vi "Session handler.vi"(0 "Loop data":T14={"Persistent"={"Last file"=path "", "Last user"="", "Users"=[]}, "Temp handle"={"Connected"=FALSE, "Temp ctrl"={"Gain (P)"=0.0, "Reset (I)"=0.0, "Rate (D)"=0.0, "Stabilization rate"=0.0, "Stabilization delta"=0.0, "Type"=enum."Lake Shore 325", "Custom temp ctrl"={"VISA resource name"=""}, "Lakeshore 325"={"VISA name"="", "Loop"=0, "Heater Range"=1, "Heater Resistance"=0, "Sample sensor"=0, "Fast sensor"=0, "Slow sensor"=0}, "Lakeshore 331"={"VISA name"="", "Loop"=1, "Heater Range"=0, "Sample sensor"=0, "Fast sensor"=0, "Slow sensor"=0}, "Lakeshore 332"={"VISA name"="", "Loop"=1, "Heater Range"=0, "Sample sensor"=0, "Fast sensor"=0, "Slow sensor"=0}, "Lakeshore 335"={"VISA name"="", "Loop"=1, "Sample sensor"=0, "Fast sensor"=0, "Slow sensor"=0, "Heater Range"=0, "Output mode"=enum."Off"}, "Lakeshore 336"={"VISA name"="", "Loop"=1, "Output mode"=enum."Off", "Max current"=1.0, "Heater resistance"=1, "Sample sensor"=1, "Slow sensor"=1, "Fast sensor"=1}}}, "Paths"={"Manual"=path "", "Settings"=path "", "Persistent"=path "", "Work dir."=path ""}, "Settings"={"MFIA"={"Address"="", "Use compensation"=TRUE, "Shut down gracefully"=FALSE}, "Temp ctrl"={"Gain (P)"=0.0, "Reset (I)"=0.0, "Rate (D)"=0.0, "Stabilization rate"=0.0, "Stabilization delta"=0.0, "Type"=enum."Lake Shore 325", "Custom temp ctrl"={"VISA resource name"=""}, "Lakeshore 325"={"VISA name"="", "Loop"=0, "Heater Range"=1, "Heater Resistance"=0, "Sample sensor"=0, "Fast sensor"=0, "Slow sensor"=0}, "Lakeshore 331"={"VISA name"="", "Loop"=1, "Heater Range"=0, "Sample sensor"=0, "Fast sensor"=0, "Slow sensor"=0}, "Lakeshore 332"={"VISA name"="", "Loop"=1, "Heater Range"=0, "Sample sensor"=0, "Fast sensor"=0, "Slow sensor"=0}, "Lakeshore 335"={"VISA name"="", "Loop"=1, "Sample sensor"=0, "Fast sensor"=0, "Slow sensor"=0, "Heater Range"=0, "Output mode"=enum."Off"}, "Lakeshore 336"={"VISA name"="", "Loop"=1, "Output mode"=enum."Off", "Max current"=1.0, "Heater resistance"=1, "Sample sensor"=1, "Slow sensor"=1, "Fast sensor"=1}}, "Source-meter"={"Type"=enum."Custom", "Custom source-meter"={"VISA resource name"=""}, "Keithley 2600"={"VISA name"="", "Ignore ID Query"=FALSE, "SMU"=enum."Channel A"}, "Keithley 2400 Series"={"VISA name"="", "Ignore ID Query"=FALSE}}, "Other"={"Enable OriginLab"=FALSE, "Reader mode"=FALSE, "Auto-save"=FALSE}, "Defaults"={"IV properties"={"T"=0.0, "Vstart"=-0.5, "Vstop"=0.5, "Vpoints"=10.0, "Settling"=0.01, "I limit"=0.1, "Log mapping"=FALSE, "Averaging"=0.0}, "CV properties"={"T"=0.0, "Vstart"=-0.5, "Vstop"=0.5, "Vpoints"=10.0, "Precision"=enum."Normal", "Test signal"=0.01, "Auto I range"=FALSE, "Test frequency"=100000.0, "I range"=-2.0, "V range"=10.0, "Log mapping"=FALSE, "Rel perm"=0.0, "Area"=0.0, "Equivalent circuit model"=0}, "DLTS properties"={"Tstart"=0.0, "Instant start"=FALSE, "Tstop"=0.0, "T rate"=0.0, "Test signal"=0.0, "Test frequency"=0.0, "Bandwidth"=0.0, "Averaging"=0.0, "Vbias"=0.0, "Vpulse"=0.0, "pulse length"=0.0, "Pulse 2"=FALSE, "Vpulse 2"=0.0, "pulse length 2"=0.0, "I range"=-2.0, "V range"=10.0, "Emission rate"=[], "Sampling rate"=0.0, "Acq. delay"=0.0, "Filter order"=0, "Equivalent circuit model"=0}, "LDLTS properties"={"T"=0.0, "Test signal"=0.0, "Test frequency"=0.0, "Bandwidth"=0.0, "Averaging"=0.0, "Vbias"=0.0, "Vpulse"=0.0, "pulse length"=0.0, "Pulse 2"=FALSE, "Vpulse 2"=0.0, "pulse length 2"=0.0, "I range"=-2.0, "V range"=10.0, "Sampling rate"=0.0, "Acq. delay"=0.0, "Sampling time"=0.0, "Filter order"=0, "Equivalent circuit model"=0}}}, "Software version"=0.0, "MFIA handle"={"ziHandle"={"handleValid"=FALSE, "Conn"=0, "Path Prefix"="", "Handle"=0, "Connected"=FALSE, "Clockbase(s)"=0.0}, "Selected device"="", "ziModHandle"={"handleValid"=FALSE, "Conn"=0, "ModHandle"=0, "moduleID"="", "Path Prefix"=""}}, "Source-meter handle"={"Connected"=FALSE, "Source-meter"={"Type"=enum."Custom", "Custom source-meter"={"VISA resource name"=""}, "Keithley 2600"={"VISA name"="", "Ignore ID Query"=FALSE, "SMU"=enum."Channel A"}, "Keithley 2400 Series"={"VISA name"="", "Ignore ID Query"=FALSE}}}} {"MFIA handle"."ziModHandle"."ModHandle" format="0x%08x"; "MFIA handle"."ziModHandle"."Conn" format="0x%08x"; "MFIA handle"."ziHandle"."Handle" format="0x%08x"; "MFIA handle"."ziHandle"."Conn" format="0x%08x"; "Settings"."Defaults"."LDLTS properties"."Equivalent circuit model" items=["Rp || Cp", "Rs + Cs", "Rs + Ls", "G B", "D Cs", "Q Cs", "D Ls", "Q Ls", "Rp || Lp", "D Cp"]; "Settings"."Defaults"."LDLTS properties"."Filter order" min=0 max=8 step=1; "Settings"."Defaults"."LDLTS properties"."Sampling rate" items=["13k"=13392.857422, "27k"=26785.714844, "54k"=53571.429687, "107k"=107142.859375]; "Settings"."Defaults"."LDLTS properties"."V range" items=["10mV"=0.01, "100mV"=0.1, "1V"=1.0, "10V"=10.0]; "Settings"."Defaults"."LDLTS properties"."I range" items=["100nA"=-7.0, "1µA"=-6.0, "10µA"=-5.0, "100µA"=-4.0, "1mA"=-3.0, "10mA"=-2.0]; "Settings"."Defaults"."DLTS properties"."Equivalent circuit model" items=["Rp || Cp", "Rs + Cs", "Rs + Ls", "G B", "D Cs", "Q Cs", "D Ls", "Q Ls", "Rp || Lp", "D Cp"]; "Settings"."Defaults"."DLTS properties"."Filter order" min=0 max=8 step=1; "Settings"."Defaults"."DLTS properties"."Sampling rate" items=["13k"=13392.857422, "27k"=26785.714844, "54k"=53571.429687, "107k"=107142.859375]; "Settings"."Defaults"."DLTS properties"."V range" items=["10mV"=0.01, "100mV"=0.1, "1V"=1.0, "10V"=10.0]; "Settings"."Defaults"."DLTS properties"."I range" items=["10mV"=0.01, "100mV"=0.1, "1V"=1.0, "10V"=10.0]; "Settings"."Defaults"."CV properties"."Equivalent circuit model" items=["Rp || Cp", "Rs + Cs", "Rs + Ls", "G B", "D Cs", "Q Cs", "D Ls", "Q Ls", "Rp || Lp", "D Cp"]; "Settings"."Defaults"."CV properties"."V range" items=["10mV"=0.01, "100mV"=0.1, "1V"=1.0, "10V"=10.0]; "Settings"."Defaults"."CV properties"."I range" items=["100nA"=-7.0, "1µA"=-6.0, "10µA"=-5.0, "100µA"=-4.0, "1mA"=-3.0, "10mA"=-2.0]; "Settings"."Defaults"."IV properties"."Settling" min=0.0 max=65535.0; "Settings"."Temp ctrl"."Lakeshore 336"."Fast sensor" items=["Sensor A", "Sensor B", "Sensor C", "Sensor D"]; "Settings"."Temp ctrl"."Lakeshore 336"."Slow sensor" items=["Sensor A", "Sensor B", "Sensor C", "Sensor D"]; "Settings"."Temp ctrl"."Lakeshore 336"."Sample sensor" items=["Sensor A", "Sensor B", "Sensor C", "Sensor D"]; "Settings"."Temp ctrl"."Lakeshore 336"."Heater resistance" items=["25 Ohm"=1, "50 Ohm"=2]; "Settings"."Temp ctrl"."Lakeshore 336"."Max current" items=["0.707 A"=0.0, "1 A"=1.0, "1.414 A"=1.414, "2 A"=2.0]; "Settings"."Temp ctrl"."Lakeshore 336"."Loop" items=["Output 1"=1, "Output 2"=2, "Output 3"=3, "Output 4"=4]; "Settings"."Temp ctrl"."Lakeshore 335"."Heater Range" items=["Off", "Low (On)", "Medium", "High"]; "Settings"."Temp ctrl"."Lakeshore 335"."Slow sensor" items=["A", "B"]; "Settings"."Temp ctrl"."Lakeshore 335"."Fast sensor" items=["A", "B"]; "Settings"."Temp ctrl"."Lakeshore 335"."Sample sensor" items=["A", "B"]; "Settings"."Temp ctrl"."Lakeshore 335"."Loop" items=["Loop 1"=1, "Loop 2"=2]; "Settings"."Temp ctrl"."Lakeshore 332"."Slow sensor" items=["A", "B"]; "Settings"."Temp ctrl"."Lakeshore 332"."Fast sensor" items=["A", "B"]; "Settings"."Temp ctrl"."Lakeshore 332"."Sample sensor" items=["A", "B"]; "Settings"."Temp ctrl"."Lakeshore 332"."Heater Range" items=["Off", "Low (0.5W)", "Med (5W)", "High (50W)"]; "Settings"."Temp ctrl"."Lakeshore 332"."Loop" items=["Loop 1", "Loop 2"]; "Settings"."Temp ctrl"."Lakeshore 331"."Slow sensor" items=["A", "B"]; "Settings"."Temp ctrl"."Lakeshore 331"."Fast sensor" items=["A", "B"]; "Settings"."Temp ctrl"."Lakeshore 331"."Sample sensor" items=["A", "B"]; "Settings"."Temp ctrl"."Lakeshore 331"."Heater Range" items=["Off", "Low (0.5W)", "Med (5W)", "High (50W)"]; "Settings"."Temp ctrl"."Lakeshore 331"."Loop" items=["Loop 1", "Loop 2"]; "Settings"."Temp ctrl"."Lakeshore 325"."Slow sensor" items=["A", "B"]; "Settings"."Temp ctrl"."Lakeshore 325"."Fast sensor" items=["A", "B"]; "Settings"."Temp ctrl"."Lakeshore 325"."Sample sensor" items=["A", "B"]; "Settings"."Temp ctrl"."Lakeshore 325"."Heater Resistance" items=["25 Ohm"=1, "50 Ohm"=2]; "Settings"."Temp ctrl"."Lakeshore 325"."Heater Range" items=["Off", "Low (loop 1) or On (loop 2)", "High (loop 1)"]; "Settings"."Temp ctrl"."Lakeshore 325"."Loop" items=["Loop 1"=1, "Loop 2"=2]; "Temp handle"."Temp ctrl"."Lakeshore 336"."Fast sensor" items=["Sensor A", "Sensor B", "Sensor C", "Sensor D"]; "Temp handle"."Temp ctrl"."Lakeshore 336"."Slow sensor" items=["Sensor A", "Sensor B", "Sensor C", "Sensor D"]; "Temp handle"."Temp ctrl"."Lakeshore 336"."Sample sensor" items=["Sensor A", "Sensor B", "Sensor C", "Sensor D"]; "Temp handle"."Temp ctrl"."Lakeshore 336"."Heater resistance" items=["25 Ohm"=1, "50 Ohm"=2]; "Temp handle"."Temp ctrl"."Lakeshore 336"."Max current" items=["0.707 A"=0.0, "1 A"=1.0, "1.414 A"=1.414, "2 A"=2.0]; "Temp handle"."Temp ctrl"."Lakeshore 336"."Loop" items=["Output 1"=1, "Output 2"=2, "Output 3"=3, "Output 4"=4]; "Temp handle"."Temp ctrl"."Lakeshore 335"."Heater Range" items=["Off", "Low (On)", "Medium", "High"]; "Temp handle"."Temp ctrl"."Lakeshore 335"."Slow sensor" items=["A", "B"]; "Temp handle"."Temp ctrl"."Lakeshore 335"."Fast sensor" items=["A", "B"]; "Temp handle"."Temp ctrl"."Lakeshore 335"."Sample sensor" items=["A", "B"]; "Temp handle"."Temp ctrl"."Lakeshore 335"."Loop" items=["Loop 1"=1, "Loop 2"=2]; "Temp handle"."Temp ctrl"."Lakeshore 332"."Slow sensor" items=["A", "B"]; "Temp handle"."Temp ctrl"."Lakeshore 332"."Fast sensor" items=["A", "B"]; "Temp handle"."Temp ctrl"."Lakeshore 332"."Sample sensor" items=["A", "B"]; "Temp handle"."Temp ctrl"."Lakeshore 332"."Heater Range" items=["Off", "Low (0.5W)", "Med (5W)", "High (50W)"]; "Temp handle"."Temp ctrl"."Lakeshore 332"."Loop" items=["Loop 1", "Loop 2"]; "Temp handle"."Temp ctrl"."Lakeshore 331"."Slow sensor" items=["A", "B"]; "Temp handle"."Temp ctrl"."Lakeshore 331"."Fast sensor" items=["A", "B"]; "Temp handle"."Temp ctrl"."Lakeshore 331"."Sample sensor" items=["A", "B"]; "Temp handle"."Temp ctrl"."Lakeshore 331"."Heater Range" items=["Off", "Low (0.5W)", "Med (5W)", "High (50W)"]; "Temp handle"."Temp ctrl"."Lakeshore 331"."Loop" items=["Loop 1", "Loop 2"]; "Temp handle"."Temp ctrl"."Lakeshore 325"."Slow sensor" items=["A", "B"]; "Temp handle"."Temp ctrl"."Lakeshore 325"."Fast sensor" items=["A", "B"]; "Temp handle"."Temp ctrl"."Lakeshore 325"."Sample sensor" items=["A", "B"]; "Temp handle"."Temp ctrl"."Lakeshore 325"."Heater Resistance" items=["25 Ohm"=1, "50 Ohm"=2]; "Temp handle"."Temp ctrl"."Lakeshore 325"."Heater Range" items=["Off", "Low (loop 1) or On (loop 2)", "High (loop 1)"]; "Temp handle"."Temp ctrl"."Lakeshore 325"."Loop" items=["Loop 1"=1, "Loop 2"=2]}, 1 "Has been propperly saved?":bool=TRUE, 5 "Session properties":T13, 7 "Workspace base":path, 9 "Actual file":path, 11 "Error In":errorcluster) -> (3 "Index out":T4 {"IV"."IV properties"."Settling" min=0.0 max=65535.0; "CV"."CV properties"."Equivalent circuit model" items=["Rp || Cp", "Rs + Cs", "Rs + Ls", "G B", "D Cs", "Q Cs", "D Ls", "Q Ls", "Rp || Lp", "D Cp"]; "CV"."CV properties"."V range" items=["10mV"=0.01, "100mV"=0.1, "1V"=1.0, "10V"=10.0]; "CV"."CV properties"."I range" items=["100nA"=-7.0, "1µA"=-6.0, "10µA"=-5.0, "100µA"=-4.0, "1mA"=-3.0, "10mA"=-2.0]; "LDLTS"."LDLTS properties"."Equivalent circuit model" items=["Rp || Cp", "Rs + Cs", "Rs + Ls", "G B", "D Cs", "Q Cs", "D Ls", "Q Ls", "Rp || Lp", "D Cp"]; "LDLTS"."LDLTS properties"."Filter order" min=0 max=8 step=1; "LDLTS"."LDLTS properties"."Sampling rate" items=["13k"=13392.857422, "27k"=26785.714844, "54k"=53571.429687, "107k"=107142.859375]; "LDLTS"."LDLTS properties"."V range" items=["10mV"=0.01, "100mV"=0.1, "1V"=1.0, "10V"=10.0]; "LDLTS"."LDLTS properties"."I range" items=["100nA"=-7.0, "1µA"=-6.0, "10µA"=-5.0, "100µA"=-4.0, "1mA"=-3.0, "10mA"=-2.0]; "Conv DLTS"."DLTS properties"."Equivalent circuit model" items=["Rp || Cp", "Rs + Cs", "Rs + Ls", "G B", "D Cs", "Q Cs", "D Ls", "Q Ls", "Rp || Lp", "D Cp"]; "Conv DLTS"."DLTS properties"."Filter order" min=0 max=8 step=1; "Conv DLTS"."DLTS properties"."Sampling rate" items=["13k"=13392.857422, "27k"=26785.714844, "54k"=53571.429687, "107k"=107142.859375]; "Conv DLTS"."DLTS properties"."V range" items=["10mV"=0.01, "100mV"=0.1, "1V"=1.0, "10V"=10.0]; "Conv DLTS"."DLTS properties"."I range" items=["10mV"=0.01, "100mV"=0.1, "1V"=1.0, "10V"=10.0]}, 4 "Loop data out":T14={"Persistent"={"Last file"=path "", "Last user"="", "Users"=[]}, "Temp handle"={"Connected"=FALSE, "Temp ctrl"={"Gain (P)"=0.0, "Reset (I)"=0.0, "Rate (D)"=0.0, "Stabilization rate"=0.0, "Stabilization delta"=0.0, "Type"=enum."Lake Shore 325", "Custom temp ctrl"={"VISA resource name"=""}, "Lakeshore 325"={"VISA name"="", "Loop"=0, "Heater Range"=1, "Heater Resistance"=0, "Sample sensor"=0, "Fast sensor"=0, "Slow sensor"=0}, "Lakeshore 331"={"VISA name"="", "Loop"=1, "Heater Range"=0, "Sample sensor"=0, "Fast sensor"=0, "Slow sensor"=0}, "Lakeshore 332"={"VISA name"="", "Loop"=1, "Heater Range"=0, "Sample sensor"=0, "Fast sensor"=0, "Slow sensor"=0}, "Lakeshore 335"={"VISA name"="", "Loop"=1, "Sample sensor"=0, "Fast sensor"=0, "Slow sensor"=0, "Heater Range"=0, "Output mode"=enum."Off"}, "Lakeshore 336"={"VISA name"="", "Loop"=1, "Output mode"=enum."Off", "Max current"=1.0, "Heater resistance"=1, "Sample sensor"=1, "Slow sensor"=1, "Fast sensor"=1}}}, "Paths"={"Manual"=path "", "Settings"=path "", "Persistent"=path "", "Work dir."=path ""}, "Settings"={"MFIA"={"Address"="", "Use compensation"=TRUE, "Shut down gracefully"=FALSE}, "Temp ctrl"={"Gain (P)"=0.0, "Reset (I)"=0.0, "Rate (D)"=0.0, "Stabilization rate"=0.0, "Stabilization delta"=0.0, "Type"=enum."Lake Shore 325", "Custom temp ctrl"={"VISA resource name"=""}, "Lakeshore 325"={"VISA name"="", "Loop"=0, "Heater Range"=1, "Heater Resistance"=0, "Sample sensor"=0, "Fast sensor"=0, "Slow sensor"=0}, "Lakeshore 331"={"VISA name"="", "Loop"=1, "Heater Range"=0, "Sample sensor"=0, "Fast sensor"=0, "Slow sensor"=0}, "Lakeshore 332"={"VISA name"="", "Loop"=1, "Heater Range"=0, "Sample sensor"=0, "Fast sensor"=0, "Slow sensor"=0}, "Lakeshore 335"={"VISA name"="", "Loop"=1, "Sample sensor"=0, "Fast sensor"=0, "Slow sensor"=0, "Heater Range"=0, "Output mode"=enum."Off"}, "Lakeshore 336"={"VISA name"="", "Loop"=1, "Output mode"=enum."Off", "Max current"=1.0, "Heater resistance"=1, "Sample sensor"=1, "Slow sensor"=1, "Fast sensor"=1}}, "Source-meter"={"Type"=enum."Custom", "Custom source-meter"={"VISA resource name"=""}, "Keithley 2600"={"VISA name"="", "Ignore ID Query"=FALSE, "SMU"=enum."Channel A"}, "Keithley 2400 Series"={"VISA name"="", "Ignore ID Query"=FALSE}}, "Other"={"Enable OriginLab"=FALSE, "Reader mode"=FALSE, "Auto-save"=FALSE}, "Defaults"={"IV properties"={"T"=0.0, "Vstart"=-0.5, "Vstop"=0.5, "Vpoints"=10.0, "Settling"=0.01, "I limit"=0.1, "Log mapping"=FALSE, "Averaging"=0.0}, "CV properties"={"T"=0.0, "Vstart"=-0.5, "Vstop"=0.5, "Vpoints"=10.0, "Precision"=enum."Normal", "Test signal"=0.01, "Auto I range"=FALSE, "Test frequency"=100000.0, "I range"=-2.0, "V range"=10.0, "Log mapping"=FALSE, "Rel perm"=0.0, "Area"=0.0, "Equivalent circuit model"=0}, "DLTS properties"={"Tstart"=0.0, "Instant start"=FALSE, "Tstop"=0.0, "T rate"=0.0, "Test signal"=0.0, "Test frequency"=0.0, "Bandwidth"=0.0, "Averaging"=0.0, "Vbias"=0.0, "Vpulse"=0.0, "pulse length"=0.0, "Pulse 2"=FALSE, "Vpulse 2"=0.0, "pulse length 2"=0.0, "I range"=-2.0, "V range"=10.0, "Emission rate"=[], "Sampling rate"=0.0, "Acq. delay"=0.0, "Filter order"=0, "Equivalent circuit model"=0}, "LDLTS properties"={"T"=0.0, "Test signal"=0.0, "Test frequency"=0.0, "Bandwidth"=0.0, "Averaging"=0.0, "Vbias"=0.0, "Vpulse"=0.0, "pulse length"=0.0, "Pulse 2"=FALSE, "Vpulse 2"=0.0, "pulse length 2"=0.0, "I range"=-2.0, "V range"=10.0, "Sampling rate"=0.0, "Acq. delay"=0.0, "Sampling time"=0.0, "Filter order"=0, "Equivalent circuit model"=0}}}, "Software version"=0.0, "MFIA handle"={"ziHandle"={"handleValid"=FALSE, "Conn"=0, "Path Prefix"="", "Handle"=0, "Connected"=FALSE, "Clockbase(s)"=0.0}, "Selected device"="", "ziModHandle"={"handleValid"=FALSE, "Conn"=0, "ModHandle"=0, "moduleID"="", "Path Prefix"=""}}, "Source-meter handle"={"Connected"=FALSE, "Source-meter"={"Type"=enum."Custom", "Custom source-meter"={"VISA resource name"=""}, "Keithley 2600"={"VISA name"="", "Ignore ID Query"=FALSE, "SMU"=enum."Channel A"}, "Keithley 2400 Series"={"VISA name"="", "Ignore ID Query"=FALSE}}}} {"MFIA handle"."ziModHandle"."ModHandle" format="0x%08x"; "MFIA handle"."ziModHandle"."Conn" format="0x%08x"; "MFIA handle"."ziHandle"."Handle" format="0x%08x"; "MFIA handle"."ziHandle"."Conn" format="0x%08x"; "Settings"."Defaults"."LDLTS properties"."Equivalent circuit model" items=["Rp || Cp", "Rs + Cs", "Rs + Ls", "G B", "D Cs", "Q Cs", "D Ls", "Q Ls", "Rp || Lp", "D Cp"]; "Settings"."Defaults"."LDLTS properties"."Filter order" min=0 max=8 step=1; "Settings"."Defaults"."LDLTS properties"."Sampling rate" items=["13k"=13392.857422, "27k"=26785.714844, "54k"=53571.429687, "107k"=107142.859375]; "Settings"."Defaults"."LDLTS properties"."V range" items=["10mV"=0.01, "100mV"=0.1, "1V"=1.0, "10V"=10.0]; "Settings"."Defaults"."LDLTS properties"."I range" items=["100nA"=-7.0, "1µA"=-6.0, "10µA"=-5.0, "100µA"=-4.0, "1mA"=-3.0, "10mA"=-2.0]; "Settings"."Defaults"."DLTS properties"."Equivalent circuit model" items=["Rp || Cp", "Rs + Cs", "Rs + Ls", "G B", "D Cs", "Q Cs", "D Ls", "Q Ls", "Rp || Lp", "D Cp"]; "Settings"."Defaults"."DLTS properties"."Filter order" min=0 max=8 step=1; "Settings"."Defaults"."DLTS properties"."Sampling rate" items=["13k"=13392.857422, "27k"=26785.714844, "54k"=53571.429687, "107k"=107142.859375]; "Settings"."Defaults"."DLTS properties"."V range" items=["10mV"=0.01, "100mV"=0.1, "1V"=1.0, "10V"=10.0]; "Settings"."Defaults"."DLTS properties"."I range" items=["10mV"=0.01, "100mV"=0.1, "1V"=1.0, "10V"=10.0]; "Settings"."Defaults"."CV properties"."Equivalent circuit model" items=["Rp || Cp", "Rs + Cs", "Rs + Ls", "G B", "D Cs", "Q Cs", "D Ls", "Q Ls", "Rp || Lp", "D Cp"]; "Settings"."Defaults"."CV properties"."V range" items=["10mV"=0.01, "100mV"=0.1, "1V"=1.0, "10V"=10.0]; "Settings"."Defaults"."CV properties"."I range" items=["100nA"=-7.0, "1µA"=-6.0, "10µA"=-5.0, "100µA"=-4.0, "1mA"=-3.0, "10mA"=-2.0]; "Settings"."Defaults"."IV properties"."Settling" min=0.0 max=65535.0; "Settings"."Temp ctrl"."Lakeshore 336"."Fast sensor" items=["Sensor A", "Sensor B", "Sensor C", "Sensor D"]; "Settings"."Temp ctrl"."Lakeshore 336"."Slow sensor" items=["Sensor A", "Sensor B", "Sensor C", "Sensor D"]; "Settings"."Temp ctrl"."Lakeshore 336"."Sample sensor" items=["Sensor A", "Sensor B", "Sensor C", "Sensor D"]; "Settings"."Temp ctrl"."Lakeshore 336"."Heater resistance" items=["25 Ohm"=1, "50 Ohm"=2]; "Settings"."Temp ctrl"."Lakeshore 336"."Max current" items=["0.707 A"=0.0, "1 A"=1.0, "1.414 A"=1.414, "2 A"=2.0]; "Settings"."Temp ctrl"."Lakeshore 336"."Loop" items=["Output 1"=1, "Output 2"=2, "Output 3"=3, "Output 4"=4]; "Settings"."Temp ctrl"."Lakeshore 335"."Heater Range" items=["Off", "Low (On)", "Medium", "High"]; "Settings"."Temp ctrl"."Lakeshore 335"."Slow sensor" items=["A", "B"]; "Settings"."Temp ctrl"."Lakeshore 335"."Fast sensor" items=["A", "B"]; "Settings"."Temp ctrl"."Lakeshore 335"."Sample sensor" items=["A", "B"]; "Settings"."Temp ctrl"."Lakeshore 335"."Loop" items=["Loop 1"=1, "Loop 2"=2]; "Settings"."Temp ctrl"."Lakeshore 332"."Slow sensor" items=["A", "B"]; "Settings"."Temp ctrl"."Lakeshore 332"."Fast sensor" items=["A", "B"]; "Settings"."Temp ctrl"."Lakeshore 332"."Sample sensor" items=["A", "B"]; "Settings"."Temp ctrl"."Lakeshore 332"."Heater Range" items=["Off", "Low (0.5W)", "Med (5W)", "High (50W)"]; "Settings"."Temp ctrl"."Lakeshore 332"."Loop" items=["Loop 1", "Loop 2"]; "Settings"."Temp ctrl"."Lakeshore 331"."Slow sensor" items=["A", "B"]; "Settings"."Temp ctrl"."Lakeshore 331"."Fast sensor" items=["A", "B"]; "Settings"."Temp ctrl"."Lakeshore 331"."Sample sensor" items=["A", "B"]; "Settings"."Temp ctrl"."Lakeshore 331"."Heater Range" items=["Off", "Low (0.5W)", "Med (5W)", "High (50W)"]; "Settings"."Temp ctrl"."Lakeshore 331"."Loop" items=["Loop 1", "Loop 2"]; "Settings"."Temp ctrl"."Lakeshore 325"."Slow sensor" items=["A", "B"]; "Settings"."Temp ctrl"."Lakeshore 325"."Fast sensor" items=["A", "B"]; "Settings"."Temp ctrl"."Lakeshore 325"."Sample sensor" items=["A", "B"]; "Settings"."Temp ctrl"."Lakeshore 325"."Heater Resistance" items=["25 Ohm"=1, "50 Ohm"=2]; "Settings"."Temp ctrl"."Lakeshore 325"."Heater Range" items=["Off", "Low (loop 1) or On (loop 2)", "High (loop 1)"]; "Settings"."Temp ctrl"."Lakeshore 325"."Loop" items=["Loop 1"=1, "Loop 2"=2]; "Temp handle"."Temp ctrl"."Lakeshore 336"."Fast sensor" items=["Sensor A", "Sensor B", "Sensor C", "Sensor D"]; "Temp handle"."Temp ctrl"."Lakeshore 336"."Slow sensor" items=["Sensor A", "Sensor B", "Sensor C", "Sensor D"]; "Temp handle"."Temp ctrl"."Lakeshore 336"."Sample sensor" items=["Sensor A", "Sensor B", "Sensor C", "Sensor D"]; "Temp handle"."Temp ctrl"."Lakeshore 336"."Heater resistance" items=["25 Ohm"=1, "50 Ohm"=2]; "Temp handle"."Temp ctrl"."Lakeshore 336"."Max current" items=["0.707 A"=0.0, "1 A"=1.0, "1.414 A"=1.414, "2 A"=2.0]; "Temp handle"."Temp ctrl"."Lakeshore 336"."Loop" items=["Output 1"=1, "Output 2"=2, "Output 3"=3, "Output 4"=4]; "Temp handle"."Temp ctrl"."Lakeshore 335"."Heater Range" items=["Off", "Low (On)", "Medium", "High"]; "Temp handle"."Temp ctrl"."Lakeshore 335"."Slow sensor" items=["A", "B"]; "Temp handle"."Temp ctrl"."Lakeshore 335"."Fast sensor" items=["A", "B"]; "Temp handle"."Temp ctrl"."Lakeshore 335"."Sample sensor" items=["A", "B"]; "Temp handle"."Temp ctrl"."Lakeshore 335"."Loop" items=["Loop 1"=1, "Loop 2"=2]; "Temp handle"."Temp ctrl"."Lakeshore 332"."Slow sensor" items=["A", "B"]; "Temp handle"."Temp ctrl"."Lakeshore 332"."Fast sensor" items=["A", "B"]; "Temp handle"."Temp ctrl"."Lakeshore 332"."Sample sensor" items=["A", "B"]; "Temp handle"."Temp ctrl"."Lakeshore 332"."Heater Range" items=["Off", "Low (0.5W)", "Med (5W)", "High (50W)"]; "Temp handle"."Temp ctrl"."Lakeshore 332"."Loop" items=["Loop 1", "Loop 2"]; "Temp handle"."Temp ctrl"."Lakeshore 331"."Slow sensor" items=["A", "B"]; "Temp handle"."Temp ctrl"."Lakeshore 331"."Fast sensor" items=["A", "B"]; "Temp handle"."Temp ctrl"."Lakeshore 331"."Sample sensor" items=["A", "B"]; "Temp handle"."Temp ctrl"."Lakeshore 331"."Heater Range" items=["Off", "Low (0.5W)", "Med (5W)", "High (50W)"]; "Temp handle"."Temp ctrl"."Lakeshore 331"."Loop" items=["Loop 1", "Loop 2"]; "Temp handle"."Temp ctrl"."Lakeshore 325"."Slow sensor" items=["A", "B"]; "Temp handle"."Temp ctrl"."Lakeshore 325"."Fast sensor" items=["A", "B"]; "Temp handle"."Temp ctrl"."Lakeshore 325"."Sample sensor" items=["A", "B"]; "Temp handle"."Temp ctrl"."Lakeshore 325"."Heater Resistance" items=["25 Ohm"=1, "50 Ohm"=2]; "Temp handle"."Temp ctrl"."Lakeshore 325"."Heater Range" items=["Off", "Low (loop 1) or On (loop 2)", "High (loop 1)"]; "Temp handle"."Temp ctrl"."Lakeshore 325"."Loop" items=["Loop 1"=1, "Loop 2"=2]}, 6 "Session properties out":T13, 8 "Workspace out":path, 10 "Actual file out":path, 15 "Error Out":errorcluster)   [LabVIEW 2019]
doc: "Handles operation in a session, displays GUI window"
uses:
  Type defs/Loop data Type Def.ctl
  Type defs/Persistent Type Def.ctl
  Type defs/Temp handle Type Def.ctl
  Type defs/Temp ctrl Type Def.ctl
  Custom devices/Custom temp ctrl settings.ctl
  Type defs/Paths Type Def.ctl
  Type defs/Settings Type Def.ctl
  Type defs/Imps Type Def.ctl
  Type defs/Source-meter Type Def.ctl
  Custom devices/Custom source-meter settings.ctl
  Type defs/Other settings Type Def.ctl
  Type defs/IV properties Type Def.ctl
  Type defs/CV properties Type Def.ctl
  Type defs/DLTS properties Type Def.ctl
  Type defs/LDLTS properties Type Def.ctl
  Type defs/MFIA handle Type Def.ctl
  <instrlib>/Zurich Instruments LabOne/Public/ziTypeHandle.ctl
  <instrlib>/Zurich Instruments LabOne/Public/Modules/ziTypeModHandle.ctl
  Type defs/Source-meter handle Type Def.ctl
  Type defs/Session properties Type Def.ctl
  Type defs/Session internal index Type Def.ctl
  Type defs/IV measurement Type Def.ctl
  Type defs/CV measurement Type Def.ctl
  Type defs/LDLTS measurement Type Def.ctl
  Type defs/cDLTS measurement Type Def.ctl
  <vilib>/Utility/error.llb/DialogType.ctl
  a9d4ef57-94a7-4ae7-bc46-4885746d2953.vi
  Parse multiple measurements to display - LDLTS.vi
  edbecbb7-eb91-4b1b-8f46-0c388df6f59b.vi
  Parse multiple measurements to display - IV.vi
  f80cbd7d-0fcc-4ac0-8a9f-9068617d6915.vi
  Parse multiple measurements to display - DLTS.vi
  6a864cb8-af1a-4f89-8bf3-16b492cd40ca.vi
  Parse multiple measurements to display - CV.vi
  Read data file (SubVI).vi
  Export single clipboard - cDLTS cluster.vi
  Export single clipboard - CV cluster.vi
  Export single clipboard - LDLTS cluster.vi
  Export single clipboard - IV cluster.vi
  Export Origin - IV.vi
  Export Origin - CV.vi
  Export Origin - cDLTS.vi
  Export Origin - LDLTS.vi
  <instrlib>/Zurich Instruments LabOne/Zurich Instruments LabOne.lvlib
panel:
  in  "Tab Control":enum32{"Tools", "Devices"}(tab)
  in  "Measurement":T1
  in  "Session":T2
  in  "Devices":T3={"MFIA"={"MFIA Connect"=FALSE, "Power"=FALSE}, "Source meter"={"SM Connect"=FALSE}, "Temperature controler"={"TC Connect"=FALSE, "Setpoint"=1.0, "Current temperature"=0.0}} {"Temperature controler"."Setpoint" min=1.0 max=800.0}
  in  "Tree":string[](tree)
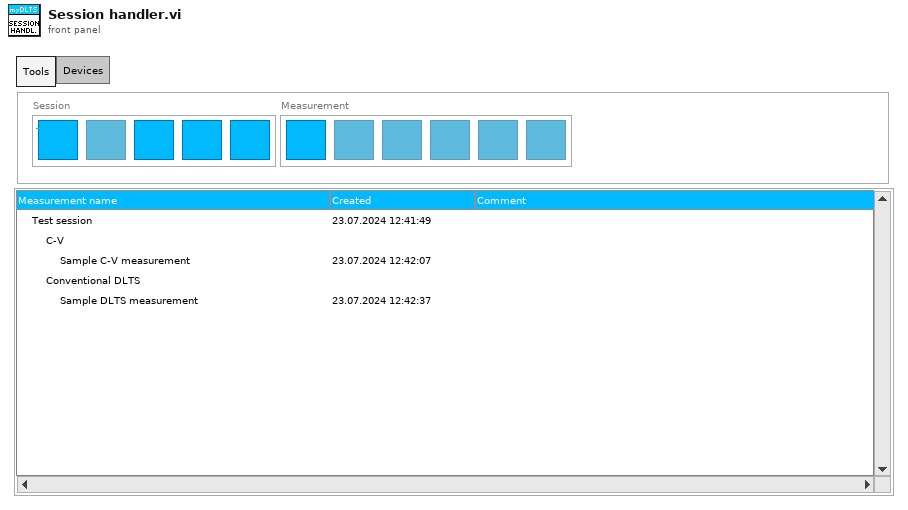
[diagram p1: front panel]
types:
  T1 = cluster{"New Measurement":bool, "View":bool, "Copy":bool, "Export":bool, "Rename":bool, "Delete":bool}
  T2 = cluster{"Information":bool, "Save":bool, "Auto Save":bool, "Help":bool, "Merge":bool}
  T3 = cluster{"MFIA":cluster{"MFIA Connect":bool, "Power":bool}, "Source meter":cluster{"SM Connect":bool}, "Temperature controler":cluster{"TC Connect":bool, "Setpoint":dbl[unit], "Current temperature":dbl[unit]}}
  T4 = typedef "Session internal index Type Def.ctl" = cluster{"IV":T5[], "CV":T7[], "LDLTS":T9[], "Conv DLTS":T11[]}
  T5 = typedef "IV measurement Type Def.ctl" = cluster{"Name":string, "Comment":string, "Time":timestamp, "Folder":path, "IV properties":T6, "GUID":string}
  T6 = typedef "IV properties Type Def.ctl" = cluster{"T":dbl[unit], "Vstart":dbl[unit], "Vstop":dbl[unit], "Vpoints":dbl, "Settling":dbl[unit], "I limit":dbl[unit], "Log mapping":bool, "Averaging":dbl}
  T7 = typedef "CV measurement Type Def.ctl" = cluster{"Name":string, "Comment":string, "Time":timestamp, "Folder":path, "CV properties":T8, "GUID":string}
  T8 = typedef "CV properties Type Def.ctl" = cluster{"T":dbl[unit], "Vstart":dbl[unit], "Vstop":dbl[unit], "Vpoints":dbl, "Precision":enum16{"Low (Fast)", "Normal", "High (Slow)"}, "Test signal":dbl[unit], "Auto I range":bool, "Test frequency":dbl[unit], "I range":dbl, "V range":dbl[unit], "Log mapping":bool, "Rel perm":dbl, "Area":dbl[unit], "Equivalent circuit model":u16}
  T9 = typedef "LDLTS measurement Type Def.ctl" = cluster{"Name":string, "Comment":string, "Time":timestamp, "Folder":path, "LDLTS properties":T10, "GUID":string}
  T10 = typedef "LDLTS properties Type Def.ctl" = cluster{"T":dbl[unit], "Test signal":dbl[unit], "Test frequency":dbl[unit], "Bandwidth":dbl[unit], "Averaging":dbl, "Vbias":dbl[unit], "Vpulse":dbl[unit], "pulse length":dbl[unit], "Pulse 2":bool, "Vpulse 2":dbl[unit], "pulse length 2":dbl[unit], "I range":dbl, "V range":dbl[unit], "Sampling rate":dbl[unit], "Acq. delay":dbl[unit], "Sampling time":dbl[unit], "Filter order":i32, "Equivalent circuit model":u16}
  T11 = typedef "cDLTS measurement Type Def.ctl" = cluster{"Name":string, "Comment":string, "Time":timestamp, "Folder":path, "DLTS properties":T12, "GUID":string}
  T12 = typedef "DLTS properties Type Def.ctl" = cluster{"Tstart":dbl[unit], "Instant start":bool, "Tstop":dbl[unit], "T rate":dbl[unit], "Test signal":dbl[unit], "Test frequency":dbl[unit], "Bandwidth":dbl[unit], "Averaging":dbl, "Vbias":dbl[unit], "Vpulse":dbl[unit], "pulse length":dbl[unit], "Pulse 2":bool, "Vpulse 2":dbl[unit], "pulse length 2":dbl[unit], "I range":dbl, "V range":dbl[unit], "Emission rate":dbl[unit][], "Sampling rate":dbl[unit], "Acq. delay":dbl[unit], "Filter order":i32, "Equivalent circuit model":u16}
  T13 = typedef "Session properties Type Def.ctl" = cluster{"Session name":string, "Comment":string, "User":string, "Software version":dbl, "Created":timestamp, "Modified":timestamp, "Binary":bool, "GUID":string}
  T14 = typedef "Loop data Type Def.ctl" = cluster{"Persistent":T15, "Temp handle":T16, "Paths":T19, "Settings":T20, "Software version":dbl, "MFIA handle":T25, "Source-meter handle":T28}
  T15 = typedef "Persistent Type Def.ctl" = cluster{"Last file":path, "Last user":string, "Users":cluster{"User":string, "Authors directory":path}[]}
  T16 = typedef "Temp handle Type Def.ctl" = cluster{"Connected":bool, "Temp ctrl":T17}
  T17 = typedef "Temp ctrl Type Def.ctl" = cluster{"Gain (P)":dbl, "Reset (I)":dbl, "Rate (D)":dbl, "Stabilization rate":dbl, "Stabilization delta":dbl, "Type":enum16{"Custom", "Lake Shore 325", "Lake Shore 331", "Lake Shore 332", "Lake Shore 335", "Lake Shore 336"}, "Custom temp ctrl":T18, "Lakeshore 325":cluster{"VISA name":refnum<visa-resource-name>, "Loop":u16, "Heater Range":u16, "Heater Resistance":u16, "Sample sensor":u16, "Fast sensor":u16, "Slow sensor":u16}, "Lakeshore 331":cluster{"VISA name":refnum<visa-resource-name>, "Loop":u16, "Heater Range":u16, "Sample sensor":u16, "Fast sensor":u16, "Slow sensor":u16}, "Lakeshore 332":cluster{"VISA name":refnum<visa-resource-name>, "Loop":u16, "Heater Range":u16, "Sample sensor":u16, "Fast sensor":u16, "Slow sensor":u16}, "Lakeshore 335":cluster{"VISA name":refnum<visa-resource-name>, "Loop":u16, "Sample sensor":u16, "Fast sensor":u16, "Slow sensor":u16, "Heater Range":u16, "Output mode":enum16{"Off", "Closed Loop PID", "Zone", "Open Loop", "Monitor Out", "Warmup Supply"}}, "Lakeshore 336":cluster{"VISA name":refnum<visa-resource-name>, "Loop":u16, "Output mode":enum16{"Off", "Closed Loop PID", "Zone", "Open Loop"}, "Max current":dbl, "Heater resistance":u16, "Sample sensor":u16, "Slow sensor":u16, "Fast sensor":u16}}
  T18 = typedef "Custom temp ctrl settings.ctl" = cluster{"VISA resource name":refnum<visa-resource-name>}
  T19 = typedef "Paths Type Def.ctl" = cluster{"Manual":path, "Settings":path, "Persistent":path, "Work dir.":path}
  T20 = typedef "Settings Type Def.ctl" = cluster{"MFIA":T21, "Temp ctrl":T17, "Source-meter":T22, "Other":T24, "Defaults":cluster{"IV properties":T6, "CV properties":T8, "DLTS properties":T12, "LDLTS properties":T10}}
  T21 = typedef "Imps Type Def.ctl" = cluster{"Address":string, "Use compensation":bool, "Shut down gracefully":bool}
  T22 = typedef "Source-meter Type Def.ctl" = cluster{"Type":enum16{"Custom", "Keithley 2600", "Keithley 2400 Series"}, "Custom source-meter":T23, "Keithley 2600":cluster{"VISA name":refnum<visa-resource-name>, "Ignore ID Query":bool, "SMU":enum16{"Channel A", "Channel B"}}, "Keithley 2400 Series":cluster{"VISA name":refnum<visa-resource-name>, "Ignore ID Query":bool}}
  T23 = typedef "Custom source-meter settings.ctl" = cluster{"VISA resource name":refnum<visa-resource-name>}
  T24 = typedef "Other settings Type Def.ctl" = cluster{"Enable OriginLab":bool, "Reader mode":bool, "Auto-save":bool}
  T25 = typedef "MFIA handle Type Def.ctl" = cluster{"ziHandle":T26, "Selected device":string, "ziModHandle":T27}
  T26 = typedef "Zurich Instruments LabOne.lvlib/ziTypeHandle.ctl" = cluster{"handleValid":bool, "Conn":u64, "Path Prefix":string, "Handle":u64, "Connected":bool, "Clockbase(s)":dbl}
  T27 = typedef "Zurich Instruments LabOne.lvlib/ziTypeModHandle.ctl" = cluster{"handleValid":bool, "Conn":u64, "ModHandle":u64, "moduleID":string, "Path Prefix":string}
  T28 = typedef "Source-meter handle Type Def.ctl" = cluster{"Connected":bool, "Source-meter":T22}
  T29 = enum8{"Enabled", "Disabled", "Disabled and Grayed Out"}
  T30 = enum32{"Invalid", "Standard", "Closed", "Hidden", "Minimized", "Maximized"}
  T31 = cluster{"Clipboard":bool, "dat":bool, "iso":bool, "Origin":bool, "Excel":bool}
  T32 = cluster{"MFIA":bool, "Temperature controller":bool, "Source meter":bool}
  T33 = typedef "DialogType.ctl" = u16
  T34 = enum16{"Left Button", "Center Button", "Right Button", "Window Close"}
  T35 = typedef "LVRectTypeDef.ctl" = cluster{"Left":i16, "Top":i16, "Right":i16, "Bottom":i16}
  T36 = enum16{"Canceled", "Clipboard", "Dat", "Iso", "Origin", "Excel"}
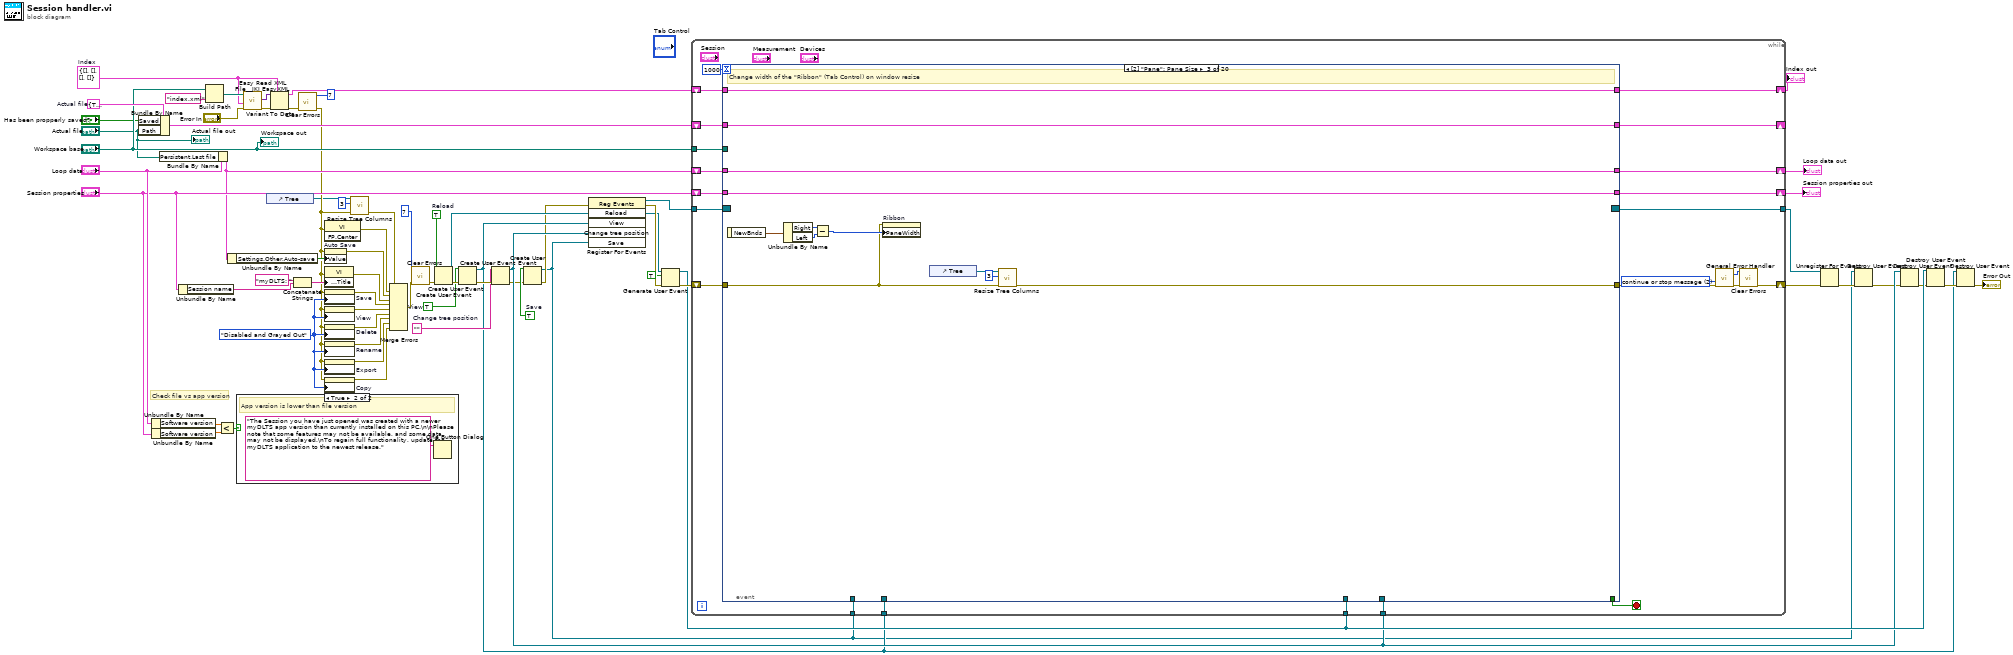
[diagram p0: block diagram]
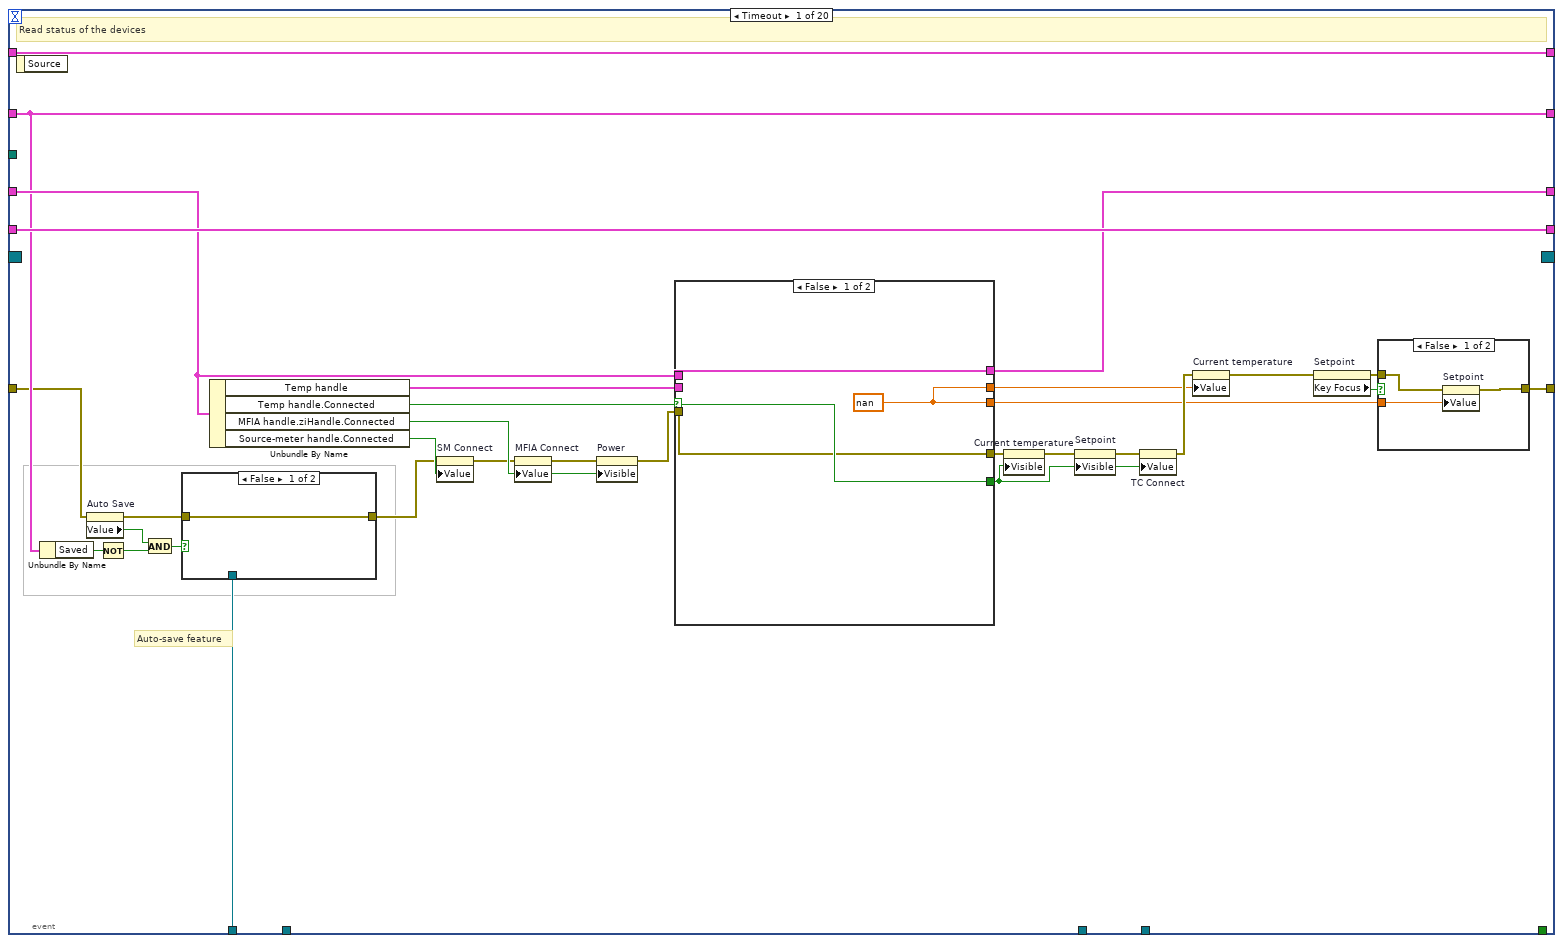
[diagram p3: hidden frame]
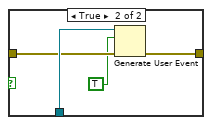
[diagram p4: hidden frame]
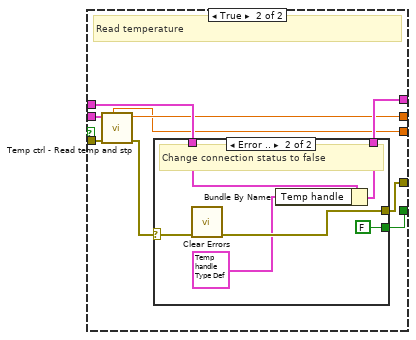
[diagram p6: hidden frame]
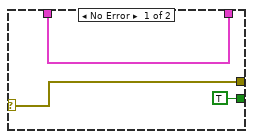
[diagram p7: hidden frame]
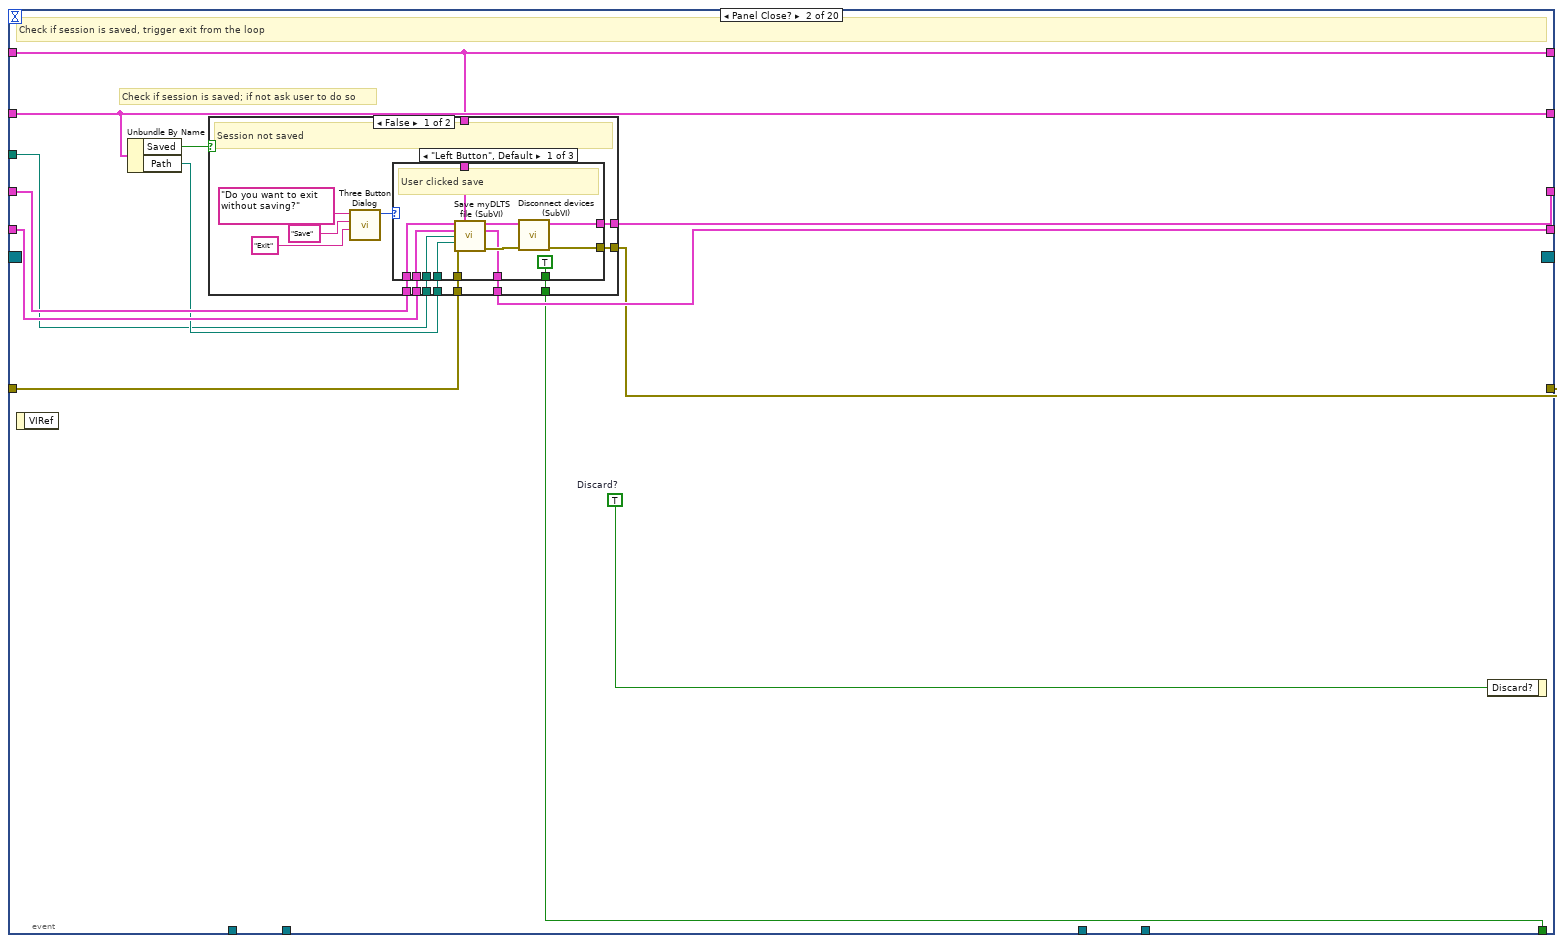
[diagram p8: hidden frame]
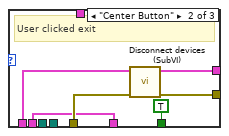
[diagram p9: hidden frame]
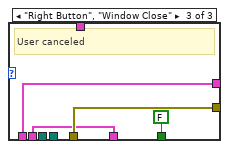
[diagram p10: hidden frame]
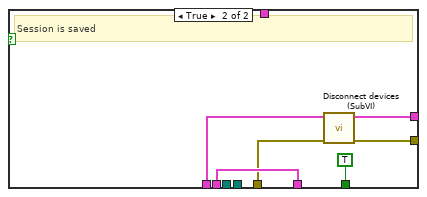
[diagram p11: hidden frame]
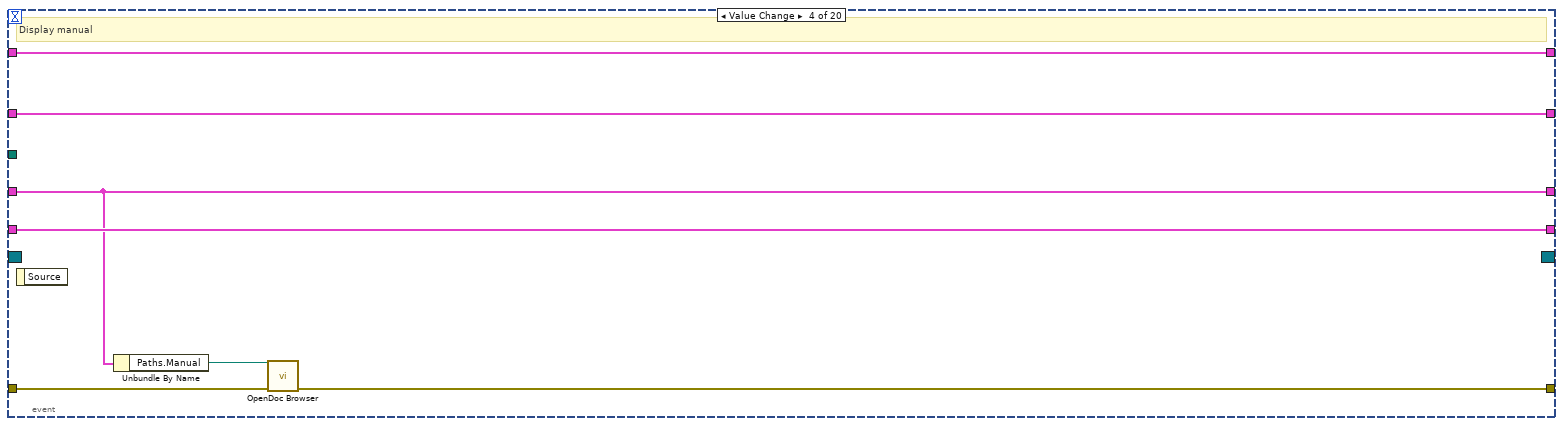
[diagram p12: hidden frame]
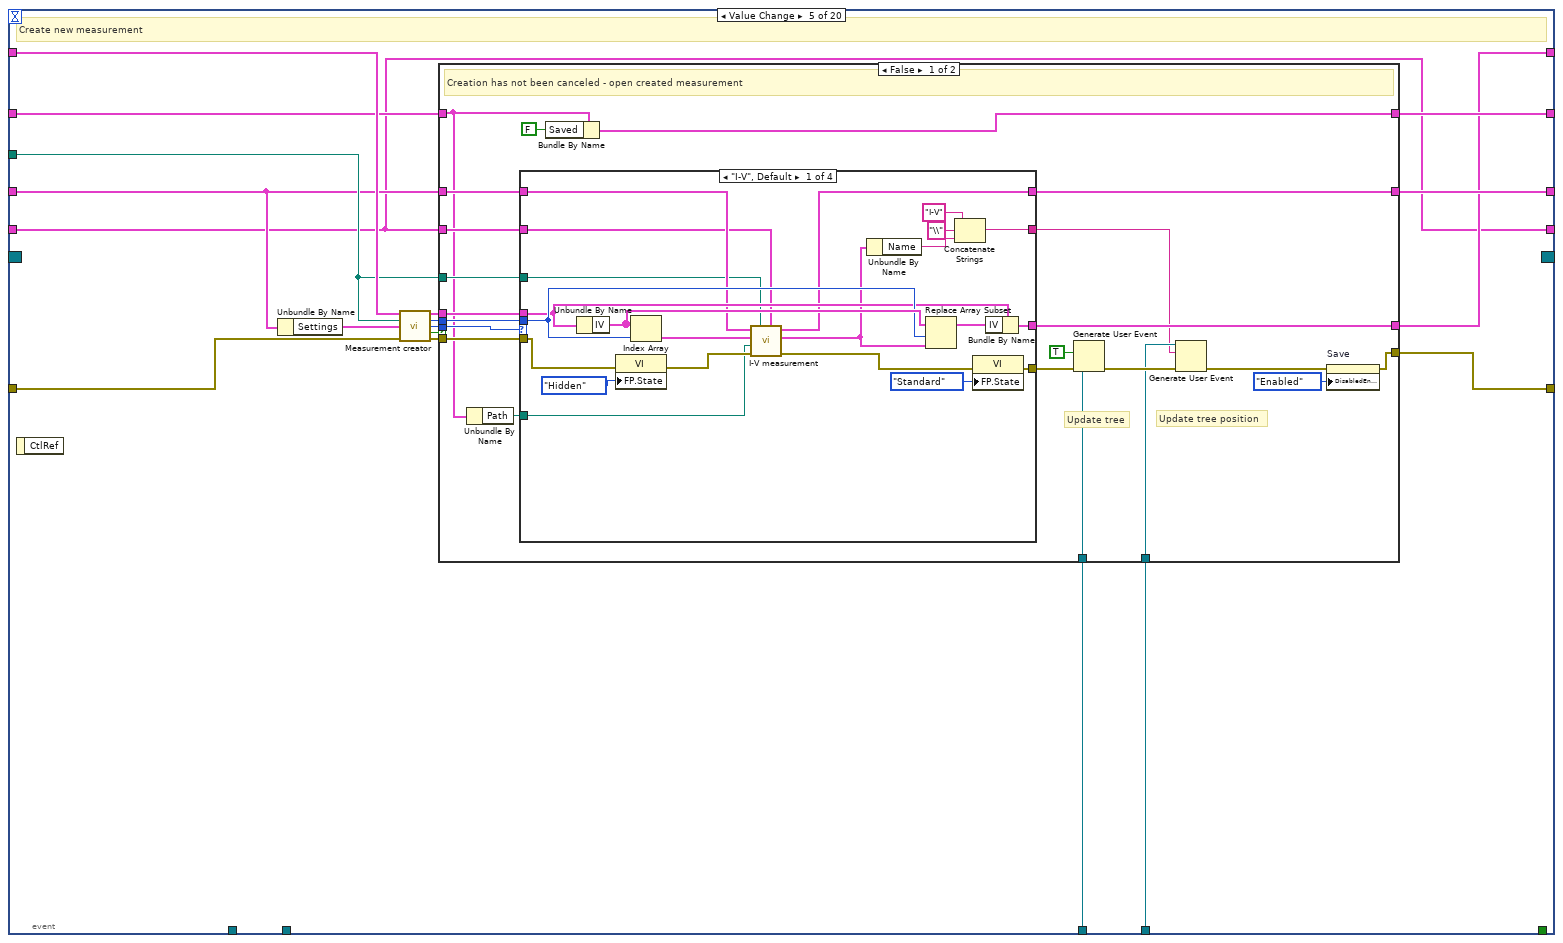
[diagram p13: hidden frame]
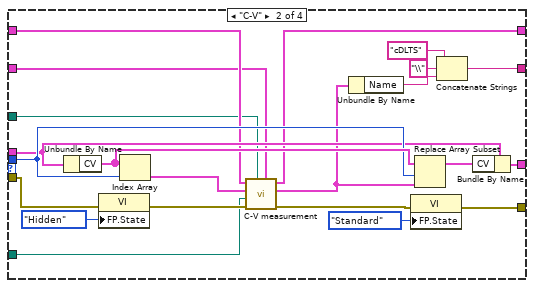
[diagram p14: hidden frame]
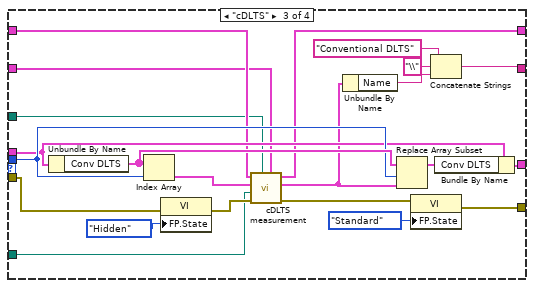
[diagram p15: hidden frame]
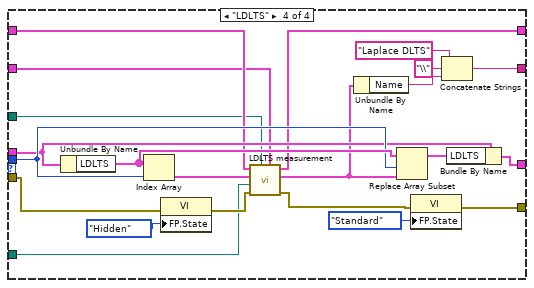
[diagram p16: hidden frame]
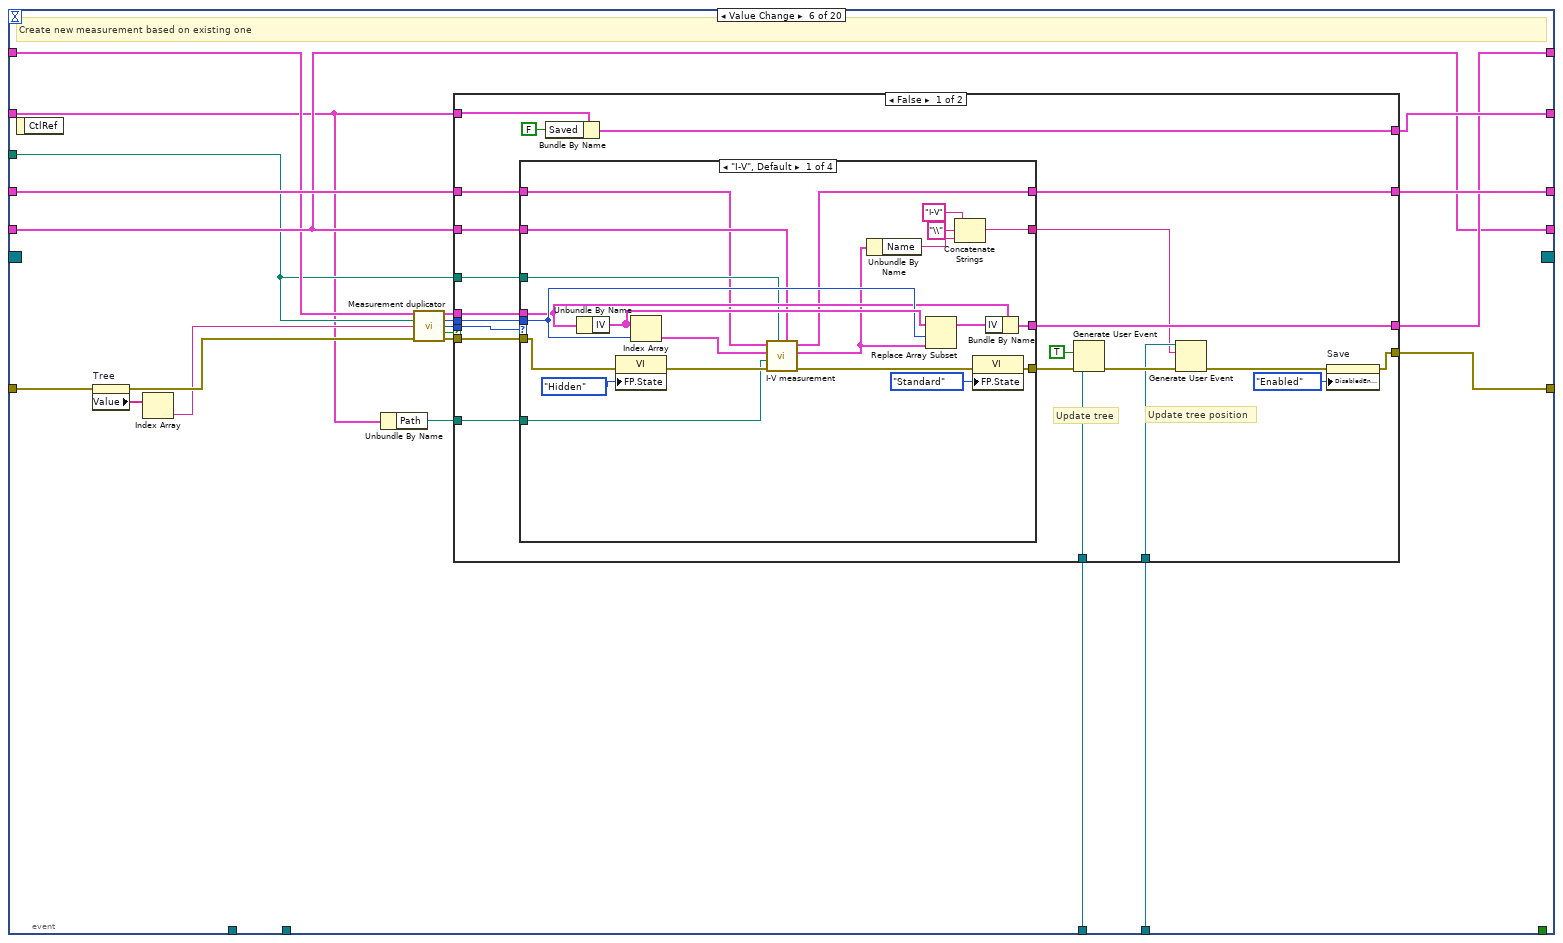
[diagram p18: hidden frame]
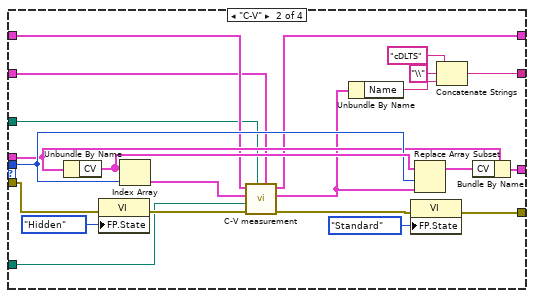
[diagram p19: hidden frame]
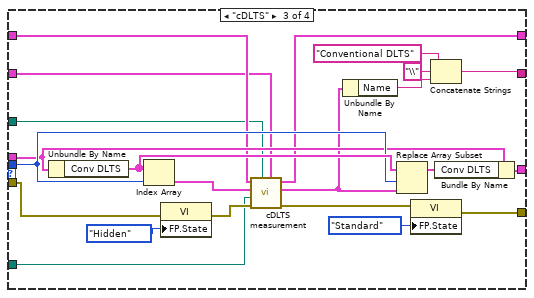
[diagram p20: hidden frame]
diagram:
  w10 = TRUE  # Save
  w28 = ""  # Change tree position
  w48 = TRUE  # View
  w21 = T29."Disabled and Grayed Out" ("Disabled")
  w43 = T4 {"IV"=[], "CV"=[], "LDLTS"=[], "Conv DLTS"=[]}  # Index
  w63 = cluster{"Saved":bool, "Path":path} {"Saved"=TRUE, "Path"=path ""}  # Actual file
  w66 = TRUE  # Reload
  # "Check file vs app version"
  n1 = Bundle By Name(cluster=w63, "Saved"="Has been propperly saved?", "Path"="Actual file") -> (w62:cluster{"Saved":bool, "Path":path})
  n2 = Unbundle By Name("Loop data") -> ("Software version"=w16:dbl)
  n3 = Unbundle By Name("Session properties") -> ("Software version"=w17:dbl)
  n4 = Bundle By Name(cluster="Loop data", "Persistent.Last file"="Actual file") -> (w12:T14)
  n5 = Unbundle By Name("Session properties") -> ("Session name"=w26:string)
  n6 = Build Path(base path="Workspace base", name or relative path="index.xml") -> (appended path=w59:path)
  n7 = Less?(x=w16, y=w17) -> (x < y?=w15:bool)
  n8 = Unbundle By Name(w12) -> ("Settings.Other.Auto-save"=w11:bool)
  n9 = case shown="True" w15 {
    frame False {
      # "App version is not lower than file verison (do nothing)"
    }
    frame True {
      # "App version is lower than file version"
      n10 = One Button Dialog(message="The Session you have just opened was created with a newer myDLTS app version than currently installed on this PC.\n\nPlease note that some features may not be available, and some data may not be displayed.\nTo regain full functionality, update the myDLTS application to the newest release.") -> ()  [unwired: 1 in, 1 out]
    }
  }
  n11 = call <vilib>:"Easy Read XML File__JKI EasyXML.vi"("error in (no error)"="Error In", "LabVIEW Data (Type)"=w43, "XML File Path"=w59) -> ("error out"=w38:errorcluster, "LabVIEW Data"=w61:variant)  [unwired: 6 in, 1 out]
  n12 = control-ref of="Tree"() -> (w1:refnum<vi>)
  n13 = Variant To Data(error in=w38, type=w43, Variant=w61) -> (data=w36:T4, error out=w37:errorcluster)
  n14 = Concatenate Strings("myDLTS: " ("string"), w26) -> (w33:string)
  n15 = call <vilib>:"Clear Errors.vi"("error in (no error)"=w37, "specific error code to clear (0: all)"=7) -> ("error out"=w2:errorcluster)  [unwired: 4 in, 1 out]
  n16 = invoke class="VI" method="FP.Center"(error in=w2) -> (error out=w25:errorcluster)  [unwired: 2 in, 2 out]
  n17 = property class="VI"(error in=w2, "Front Panel.Title"=w33) -> (error out=w34:errorcluster)  [unwired: 1 in, 1 out]
  n18 = property on="Save" class="Bool"(error in=w2, "DisabledEnum"=w21) -> (error out=w42:errorcluster)  [unwired: 1 in, 1 out]
  n19 = property on="View" class="Bool"(error in=w2, "DisabledEnum"=w21) -> (error out=w41:errorcluster)  [unwired: 1 in, 1 out]
  n20 = property on="Delete" class="Bool"(error in=w2, "DisabledEnum"=w21) -> (error out=w40:errorcluster)  [unwired: 1 in, 1 out]
  n21 = property on="Rename" class="Bool"(error in=w2, "DisabledEnum"=w21) -> (error out=w23:errorcluster)  [unwired: 1 in, 1 out]
  n22 = property on="Export" class="Bool"(error in=w2, "DisabledEnum"=w21) -> (error out=w31:errorcluster)  [unwired: 1 in, 1 out]
  n23 = property on="Copy" class="Bool"(error in=w2, "DisabledEnum"=w21) -> (error out=w20:errorcluster)  [unwired: 1 in, 1 out]
  n24 = property on="Auto Save" class="Bool (strict)"(error in=w2, "Value"=w11) -> (error out=w13:errorcluster)  [unwired: 1 in, 1 out]
  n25 = call "Resize Tree Columns.vi"("error in"=w2, "Number of columns"=3, "TreeControl ref in"=w1) -> ("error out"=w3:errorcluster)  [unwired: 8 in]
  n26 = Merge Errors(w3, w25, w13, w34, w42, w41, w40, w23, w31, w20) -> (w50:errorcluster)
  n27 = call <vilib>:"Clear Errors.vi"("error in (no error)"=w50, "specific error code to clear (0: all)"=7) -> ("error out"=w52:errorcluster)  [unwired: 4 in, 1 out]
  n28 = Create User Event(user event datatype=w66, error in=w52) -> (user event=w47:refnum<user-event>, error out=w49:errorcluster)
  n29 = Create User Event(user event datatype=w48, error in=w49) -> (user event=w22:refnum<user-event>, error out=w29:errorcluster)
  n30 = Create User Event(user event datatype=w28, error in=w29) -> (user event=w27:refnum<user-event>, error out=w9:errorcluster)
  n31 = Create User Event(user event datatype=w10, error in=w9) -> (user event=w5:refnum<user-event>, error out=w8:errorcluster)
  n32 = register-events(error in=w8, w47, w22, w27, w5) -> (reference out=w68:refnum<event-registration>, error out=w67:errorcluster)  [unwired: 1 in]
  n33 = Generate User Event(user event=w47, event data cluster=TRUE ("event data"), error in=w67) -> (user event out=w35:refnum<user-event>, error out=w64:errorcluster)  [unwired: 1 in]
  n34 = while {
    tunnel: w68 -> [w91]
    shift-right: [w83] -> w57
    shift-left: w12 -> [w87]
    shift-right: [w80] -> w56
    shift-left: "Session properties" -> [w86]
    shift-right: [w71] -> w54
    shift-left: w64 -> [w85]
    shift-right: [w82] -> _
    shift-left: w62 -> [w90]
    tunnel: "Workspace base" -> [w88]
    shift-right: [w81] -> w44
    shift-left: w36 -> [w89]
    tunnel: [w84] -> w55
    tunnel: w22 -> [w79]
    tunnel: w35 -> [w78]
    tunnel: w27 -> [w76]
    tunnel: w5 -> [w70]
    stop <- w92 stop-if-true
    w74 = T33 2 items=["no dialog", "OK message", "continue or stop message", "OK message + warnings", "continue/stop + warnings"] ("type of dialog (OK msg:1)")
    n35 = event shown="[2] \"Pane\": Pane Size" {
      selector: w91 -> [_ _ _ _ _ _ _ _ _ _ _ _ _ _ _ _ _ _ _ _]
      dyn-events: [_ _ _ _ _ _ _ _ _ _ _ _ _ _ _ _ _ _ _ _] -> w84
      timeout: 1000 -> [_ _ _ _ _ _ _ _ _ _ _ _ _ _ _ _ _ _ _ _]
      tunnel: [_ w155 _ _ _ _ _ _ _ _ _ _ _ _ _ _ _ _ _ _] -> w92
      tunnel: w90 -> [w99 w166 w219 w223 w239 w362 w500 w740 w877 w1030 w1041 w1071 w1098 w1249 w1267 w1287 w1305 w1442 w1464 w1473]
      tunnel: w89 -> [w122 w165 w220 w222 w246 w368 w513 w743 w880 w1038 w1048 w1069 w1097 w1248 w1266 w1288 w1304 w1441 w1463 w1472]
      tunnel: w88 -> [_ w159 _ _ w236 w367 w505 w732 _ _ w1051 w1074 _ _ _ _ w1303 _ _ _]
      tunnel: w87 -> [w118 w162 w218 w224 w231 w375 w504 w745 w882 w1039 w1050 w1068 w1099 w1250 w1268 w1286 w1301 w1431 w1458 w1468]
      tunnel: w86 -> [w123 w161 w217 w225 w229 w374 w501 w746 w883 w1035 w1049 w1067 w1096 w1251 w1269 w1284 w1300 w1440 w1462 w1471]
      tunnel: w85 -> [w95 w158 w213 w228 w245 w365 w517 w741 w878 w1037 w1052 w1075 w1102 w1247 w1265 w1283 w1306 w1429 w1460 w1470]
      tunnel: [w106 w156 w212 w226 w233 w377 w514 w737 w873 w1036 w1043 w1063 w1077 w1246 w1261 w1280 w1302 w1428 w1459 w1469] -> w75
      tunnel: [w117 w157 w218 w224 w235 w379 w503 w745 w882 w1039 w1050 w1066 w1099 w1250 w1268 w1286 w1301 w1430 w1458 w1467] -> w83
      tunnel: [w99 w166 w219 w223 w237 w380 w509 w739 w876 w1028 w1040 w1070 w1098 w1249 w1267 w1287 w1305 w1442 w1464 w1473] -> w82
      tunnel: [w122 w165 w220 w222 w234 w378 w512 w742 w879 w1038 w1046 w1069 w1097 w1248 w1266 w1288 w1304 w1441 w1463 w1472] -> w81
      tunnel: [w123 w163 w217 w225 w229 w374 w501 w746 w883 w1034 w1047 w1065 w1096 w1251 w1269 w1284 w1300 w1440 w1462 w1471] -> w80
      tunnel: w79 -> [_ _ _ _ _ _ _ _ _ _ _ _ _ w1245 _ _ _ _ _ _]
      tunnel: w78 -> [_ _ _ _ w238 w381 w506 w730 w868 _ w1042 _ _ _ _ _ _ _ _ _]
      tunnel: w76 -> [_ _ _ _ w232 w376 _ _ _ _ _ _ _ _ _ _ _ _ _ _]
      tunnel: w70 -> [w93 _ _ _ _ _ _ _ _ _ _ _ _ _ _ _ _ _ _ _]
      event Timeout {
        # "Auto-save feature"
        # "Read status of the devices"
        n36 = event-data() -> ()  [unwired: 1 in, 1 out]
        n37 = Unbundle By Name(w99) -> ("Saved"=w98:bool)
        n38 = property on="Auto Save" class="Bool (strict)"(error in=w95) -> (error out=w94:errorcluster, "Value"=w96:bool)  [unwired: 1 in, 1 out]
        n39 = Not(x=w98) -> (.not. x?=w97:bool)
        n40 = And(x=w96, y=w97) -> (x .and. y?=w100:bool)
        n41 = case shown="False" w100 {
          tunnel: w94 -> [w124 w127]
          tunnel: [w124 w126] -> w101
          tunnel: w93 -> [_ w128]
          frame False {
          }
          frame True {
            n42 = Generate User Event(user event=w128, event data cluster=TRUE ("event data"), error in=w127) -> (error out=w126:errorcluster)  [unwired: 1 in, 1 out]
          }
        }
        n43 = Unbundle By Name(w118) -> ("Temp handle"=w121:T16, "Temp handle.Connected"=w120:bool, "MFIA handle.ziHandle.Connected"=w111:bool, "Source-meter handle.Connected"=w103:bool)
        n44 = property on="SM Connect" class="Bool (strict)"(error in=w101, "Value"=w103) -> (error out=w102:errorcluster)  [unwired: 1 in, 1 out]
        n45 = property on="MFIA Connect" class="Bool (strict)"(error in=w102, "Value"=w111) -> (error out=w113:errorcluster)  [unwired: 1 in, 1 out]
        n46 = property on="Power" class="Bool"(error in=w113, "Visible"=w111) -> (error out=w112:errorcluster)  [unwired: 1 in, 1 out]
        n47 = case shown="False" w120 {
          selector: w120 -> [w136 _]
          tunnel: w121 -> [_ w140]
          tunnel: w112 -> [w135 w141]
          tunnel: [w133 w138] -> w105
          tunnel: [w135 w145] -> w119
          tunnel: w118 -> [w134 w144]
          tunnel: [w134 w143] -> w117
          tunnel: [w136 w142] -> w115
          tunnel: [w133 w137] -> w104
          frame False {
            w133 = dbl[unit] nan ("Sensor Data")
          }
          frame True {
            # "Read temperature"
            n48 = call "Temp ctrl - Read temp and stp.vi"("Error In"=w141, "Temp handle"=w140) -> ("Error Out"=w139:errorcluster, "Sample temperature"=w138:dbl[unit], "Setpoint"=w137:dbl[unit])  [unwired: 2 in, 2 out]
            n49 = case shown="Error .." w139 {
              selector: w139 -> [w148 w153]
              tunnel: [w148 w154] -> w145
              tunnel: w144 -> [w147 w152]
              tunnel: [w147 w150] -> w143
              tunnel: [TRUE FALSE] -> w142
              frame No Error {
              }
              frame Error {
                # "Change connection status to false"
                n50 = call <vilib>:"Clear Errors.vi"("error in (no error)"=w153) -> ("error out"=w154:errorcluster)  [unwired: 5 in, 1 out]
                n51 = Bundle By Name(cluster=w152, "Temp handle"=T16 {"Connected"=FALSE, "Temp ctrl"={"Gain (P)"=0.0, "Reset (I)"=0.0, "Rate (D)"=0.0, "Stabilization rate"=0.0, "Stabilization delta"=0.0, "Type"=enum."Lake Shore 325", "Custom temp ctrl"={"VISA resource name"=""}, "Lakeshore 325"={"VISA name"="", "Loop"=0, "Heater Range"=1, "Heater Resistance"=0, "Sample sensor"=0, "Fast sensor"=0, "Slow sensor"=0}, "Lakeshore 331"={"VISA name"="", "Loop"=1, "Heater Range"=0, "Sample sensor"=0, "Fast sensor"=0, "Slow sensor"=0}, "Lakeshore 332"={"VISA name"="", "Loop"=1, "Heater Range"=0, "Sample sensor"=0, "Fast sensor"=0, "Slow sensor"=0}, "Lakeshore 335"={"VISA name"="", "Loop"=1, "Sample sensor"=0, "Fast sensor"=0, "Slow sensor"=0, "Heater Range"=0, "Output mode"=enum."Off"}, "Lakeshore 336"={"VISA name"="", "Loop"=1, "Output mode"=enum."Off", "Max current"=1.0, "Heater resistance"=1, "Sample sensor"=1, "Slow sensor"=1, "Fast sensor"=1}}}) -> (w150:T14)
              }
            }
          }
        }
        n52 = property on="Current temperature" class="DigNum (strict)"(error in=w119, "Visible"=w115) -> (error out=w116:errorcluster)  [unwired: 1 in, 1 out]
        n53 = property on="Setpoint" class="DigNum (strict)"(error in=w116, "Visible"=w115) -> (error out=w114:errorcluster)  [unwired: 1 in, 1 out]
        n54 = property on="TC Connect" class="Bool (strict)"(error in=w114, "Value"=w115) -> (error out=w110:errorcluster)  [unwired: 1 in, 1 out]
        n55 = property on="Current temperature" class="DigNum (strict)"(error in=w110, "Value"=w105) -> (error out=w109:errorcluster)  [unwired: 1 in, 1 out]
        n56 = property on="Setpoint" class="DigNum (strict)"(error in=w109) -> (error out=w108:errorcluster, "Key Focus"=w107:bool)  [unwired: 1 in, 1 out]
        n57 = case shown="False" w107 {
          tunnel: w104 -> [w131 _]
          tunnel: w108 -> [w130 w132]
          tunnel: [w129 w132] -> w106
          frame False {
            n58 = property on="Setpoint" class="DigNum (strict)"(error in=w130, "Value"=w131) -> (error out=w129:errorcluster)  [unwired: 1 in, 1 out]
          }
          frame True {
          }
        }
      }
      event Panel Close? {
        w167 = TRUE  # Discard?
        # "Check if session is saved; if not ask user to do so"
        # "Check if session is saved, trigger exit from the loop"
        n59 = event-data() -> ()  [unwired: 1 in, 1 out]
        n60 = Unbundle By Name(w166) -> ("Saved"=w164:bool, "Path"=w160:path)
        n61 = case shown="False" w164 {
          tunnel: w165 -> [w181 _]
          tunnel: [w176 w206] -> w163
          tunnel: w162 -> [w175 w205]
          tunnel: w161 -> [w174 w206]
          tunnel: w160 -> [w173 _]
          tunnel: w159 -> [w172 _]
          tunnel: w158 -> [w171 w204]
          tunnel: [w170 w208] -> w156
          tunnel: [w169 w209] -> w157
          tunnel: [w168 TRUE] -> w155
          frame False {
            # "Session not saved"
            n62 = call <vilib>:"Three Button Dialog.vi"("Center Button Text (\"No\")"="Exit" ("Center Button Text (\"No\")"), "Left Button Text (\"Yes\")"="Save" ("Left Button Text (\"Yes\")"), "message"="Do you want to exit without saving?") -> ("Which Button?"=w177:T34)  [unwired: 8 in]
            n63 = case shown="\"Left Button\", Default" w177 {
              tunnel: w181 -> [w193 _ _]
              tunnel: [w190 w195 w201] -> w176
              tunnel: w175 -> [w189 w196 w203]
              tunnel: w174 -> [w188 w195 w201]
              tunnel: w173 -> [w187 _ _]
              tunnel: w172 -> [w186 _ _]
              tunnel: w171 -> [w185 w197 w202]
              tunnel: [w184 w199 w202] -> w170
              tunnel: [w183 w198 w203] -> w169
              tunnel: [TRUE TRUE FALSE] -> w168
              frame "Left Button", Default {
                # "User clicked save"
                n64 = call "Save myDLTS file (SubVI).vi"("Loop data in"=w189, "Index"=w193, "Session properties"=w188, "Workspace path"=w186, "File"=w187, "Error In"=w185) -> ("Loop data out"=w191:T14, "Session properties out"=w190:T13, "Error  out"=w192:errorcluster)  [unwired: 5 in, 2 out]
                n65 = call "Disconnect devices (SubVI).vi"("error in (no error)"=w192, "Loop data"=w191) -> ("Error Out"=w184:errorcluster, "Loop data out"=w183:T14)  [unwired: 8 in]
              }
              frame "Center Button" {
                # "User clicked exit"
                n66 = call "Disconnect devices (SubVI).vi"("error in (no error)"=w197, "Loop data"=w196) -> ("Error Out"=w199:errorcluster, "Loop data out"=w198:T14)  [unwired: 8 in]
              }
              frame "Right Button", "Window Close" {
                # "User canceled"
              }
            }
          }
          frame True {
            # "Session is saved"
            n67 = call "Disconnect devices (SubVI).vi"("error in (no error)"=w204, "Loop data"=w205) -> ("Error Out"=w208:errorcluster, "Loop data out"=w209:T14)  [unwired: 8 in]
          }
        }
        n68 = event-data("Discard?"=w167) -> ()  [unwired: 1 in, 1 out]
      }
      event Pane Size {
        # "Change width of the \"Ribbon\" (Tab Control) on window resize"
        n69 = event-data() -> ("NewBnds"=w221:T35)  [unwired: 1 in]
        n70 = Unbundle By Name(w221) -> ("Right"=w216:i16, "Left"=w215:i16)
        n71 = Subtract(x=w216, y=w215) -> (x-y=w214:i16)
        n72 = property on="Ribbon" class="TabCtl (strict)"(error in=w213, "PaneWidth"=w214) -> ()  [unwired: 1 in, 2 out]
        n73 = control-ref of="Tree"() -> (w211:refnum<vi>)
        n74 = call "Resize Tree Columns.vi"("error in"=w213, "Number of columns"=3, "TreeControl ref in"=w211) -> ("error out"=w212:errorcluster)  [unwired: 8 in]
      }
      event "Session.Help": Value Change {
        # "Display manual"
        n75 = event-data() -> ()  [unwired: 1 in, 1 out]
        n76 = Unbundle By Name(w224) -> ("Paths.Manual"=w227:path)
        n77 = call "OpenDoc Browser.vi"("error in (no error)"=w228, "File"=w227) -> ("error out"=w226:errorcluster)  [unwired: 9 in]
      }
      event "Measurement.New Measurement": Value Change {
        # "Create new measurement"
        n78 = event-data() -> ()  [unwired: 1 in, 1 out]
        n79 = Unbundle By Name(w231) -> ("Settings"=w230:T20)
        n80 = call "Measurement creator.vi"("Index in"=w246, "Workspace"=w236, "Settings"=w230, "error in (no error)"=w245) -> ("Index out"=w240:T4, "ID"=w241:i32, "Type"=w242:enum16{"I-V", "C-V", "cDLTS", "LDLTS"}, "Canceled"=w244:bool, "error out"=w243:errorcluster)  [unwired: 7 in]
        n81 = case shown="False" w244 {
          tunnel: w243 -> [w266 w359]
          tunnel: w242 -> [w267 _]
          tunnel: w241 -> [w264 _]
          tunnel: w240 -> [w265 w360]
          tunnel: w239 -> [w248 w358]
          tunnel: [w263 w360] -> w234
          tunnel: [w257 w359] -> w233
          tunnel: w238 -> [w260 _]
          tunnel: [w259 w358] -> w237
          tunnel: w236 -> [w256 _]
          tunnel: w231 -> [w255 w357]
          tunnel: [w254 w357] -> w235
          tunnel: w232 -> [w251 _]
          tunnel: w229 -> [w249 _]
          frame False {
            # "Update tree position"
            # "Update tree"
            # "Creation has not been canceled - open created measurement"
            n82 = Unbundle By Name(w248) -> ("Path"=w247:path)
            n83 = case shown="\"I-V\", Default" w267 {
              tunnel: w266 -> [w290 w312 w334 w356]
              tunnel: w265 -> [w286 w308 w330 w352]
              tunnel: w264 -> [w287 w309 w331 w353]
              tunnel: [w284 w306 w328 w350] -> w261
              tunnel: [w283 w305 w327 w349] -> w263
              tunnel: w256 -> [w274 w298 w316 w336]
              tunnel: w255 -> [w276 w300 w318 w339]
              tunnel: [w271 w299 w317 w338] -> w254
              tunnel: [w278 w294 w322 w344] -> w250
              tunnel: w249 -> [w270 w292 w314 w337]
              tunnel: w247 -> [w269 w291 w313 w335]
              frame "I-V", Default {
                n84 = Unbundle By Name(w286) -> ("IV"=w288:T5[])
                n85 = property class="VI"(error in=w290, "FP.State"=T30."Hidden" ("Front Panel Window:State")) -> (error out=w277:errorcluster)  [unwired: 1 in, 1 out]
                n86 = Index Array(array=w288, index=w287) -> (element=w275:T5)
                n87 = call "I-V measurement.vi"("Session properties"=w270, "Workspace"=w274, "Error In"=w277, "myDLTS file path"=w269, "IV measurement"=w275, "Loop data"=w276) -> ("Error Out"=w273:errorcluster, "IV measurement out"=w272:T5, "Loop data out"=w271:T14)  [unwired: 2 in, 1 out]
                n88 = Unbundle By Name(w272) -> ("Name"=w281:string)
                n89 = Replace Array Subset(array=w288, new element=w272, index=w287) -> (w285:T5[])
                n90 = Concatenate Strings("I-V" ("string"), "\\" ("string"), w281) -> (w278:string)
                n91 = property class="VI"(error in=w273, "FP.State"=T30."Standard" ("Front Panel Window:State")) -> (error out=w284:errorcluster)  [unwired: 1 in, 1 out]
                n92 = Bundle By Name(cluster=w286, "IV"=w285) -> (w283:T4)
              }
              frame "C-V" {
                n93 = Unbundle By Name(w308) -> ("CV"=w310:T7[])
                n94 = property class="VI"(error in=w312, "FP.State"=T30."Hidden" ("Front Panel Window:State")) -> (error out=w303:errorcluster)  [unwired: 1 in, 1 out]
                n95 = Index Array(array=w310, index=w309) -> (element=w302:T7)
                n96 = call "C-V measurement.vi"("Session properties"=w292, "Workspace"=w298, "Error In"=w303, "myDLTS file path"=w291, "CV measurement"=w302, "Loop data"=w300) -> ("Error Out"=w301:errorcluster, "CV measurement out"=w293:T7, "Loop data out"=w299:T14)  [unwired: 2 in, 1 out]
                n97 = Unbundle By Name(w293) -> ("Name"=w297:string)
                n98 = property class="VI"(error in=w301, "FP.State"=T30."Standard" ("Front Panel Window:State")) -> (error out=w306:errorcluster)  [unwired: 1 in, 1 out]
                n99 = Replace Array Subset(array=w310, new element=w293, index=w309) -> (w307:T7[])
                n100 = Concatenate Strings("cDLTS" ("string"), "\\" ("string"), w297) -> (w294:string)
                n101 = Bundle By Name(cluster=w308, "CV"=w307) -> (w305:T4)
              }
              frame "cDLTS" {
                n102 = Unbundle By Name(w330) -> ("Conv DLTS"=w332:T11[])
                n103 = Index Array(array=w332, index=w331) -> (element=w315:T11)
                n104 = property class="VI"(error in=w334, "FP.State"=T30."Hidden" ("Front Panel Window:State")) -> (error out=w321:errorcluster)  [unwired: 1 in, 1 out]
                n105 = call "cDLTS measurement.vi"("Session properties"=w314, "Workspace"=w316, "Error In"=w321, "myDLTS file path"=w313, "cDLTS measurement"=w315, "Loop data"=w318) -> ("Error Out"=w320:errorcluster, "cDLTS measurement out"=w319:T11, "Loop data out"=w317:T14)  [unwired: 2 in, 1 out]
                n106 = Unbundle By Name(w319) -> ("Name"=w325:string)
                n107 = Replace Array Subset(array=w332, new element=w319, index=w331) -> (w329:T11[])
                n108 = property class="VI"(error in=w320, "FP.State"=T30."Standard" ("Front Panel Window:State")) -> (error out=w328:errorcluster)  [unwired: 1 in, 1 out]
                n109 = Concatenate Strings("Conventional DLTS" ("string"), "\\" ("string"), w325) -> (w322:string)
                n110 = Bundle By Name(cluster=w330, "Conv DLTS"=w329) -> (w327:T4)
              }
              frame "LDLTS" {
                n111 = Unbundle By Name(w352) -> ("LDLTS"=w354:T9[])
                n112 = Index Array(array=w354, index=w353) -> (element=w341:T9)
                n113 = property class="VI"(error in=w356, "FP.State"=T30."Hidden" ("Front Panel Window:State")) -> (error out=w343:errorcluster)  [unwired: 1 in, 1 out]
                n114 = call "LDLTS measurement.vi"("Session properties"=w337, "Workspace"=w336, "Error In"=w343, "myDLTS file path"=w335, "LDLTS measurement"=w341, "Loop data"=w339) -> ("Error Out"=w342:errorcluster, "LDLTS measurement out"=w340:T9, "Loop data out"=w338:T14)  [unwired: 2 in, 1 out]
                n115 = Unbundle By Name(w340) -> ("Name"=w347:string)
                n116 = Replace Array Subset(array=w354, new element=w340, index=w353) -> (w351:T9[])
                n117 = property class="VI"(error in=w342, "FP.State"=T30."Standard" ("Front Panel Window:State")) -> (error out=w350:errorcluster)  [unwired: 1 in, 1 out]
                n118 = Concatenate Strings("Laplace DLTS" ("string"), "\\" ("string"), w347) -> (w344:string)
                n119 = Bundle By Name(cluster=w352, "LDLTS"=w351) -> (w349:T4)
              }
            }
            n120 = Bundle By Name(cluster=w248, "Saved"=FALSE) -> (w259:cluster{"Saved":bool, "Path":path})
            n121 = Generate User Event(user event=w260, event data cluster=TRUE ("event data"), error in=w261) -> (error out=w253:errorcluster)  [unwired: 1 in, 1 out]
            n122 = Generate User Event(user event=w251, event data cluster=w250, error in=w253) -> (error out=w252:errorcluster)  [unwired: 1 in, 1 out]
            n123 = property on="Save" class="Bool"(error in=w252, "DisabledEnum"=T29."Enabled" ("Disabled")) -> (error out=w257:errorcluster)  [unwired: 1 in, 1 out]
          }
          frame True {
            # "Creation has been canceled"
          }
        }
      }
      event "Measurement.Copy": Value Change {
        # "Create new measurement based on existing one"
        n124 = event-data() -> ()  [unwired: 1 in, 1 out]
        n125 = property on="Tree" class="Tree (strict)"(error in=w365) -> (error out=w366:errorcluster, "Value"=w364:string[])  [unwired: 1 in, 1 out]
        n126 = Index Array(array=w364) -> (element=w363:string)  [unwired: 1 in]
        n127 = Unbundle By Name(w362) -> ("Path"=w361:path)
        n128 = call "Measurement duplicator.vi"("Index in"=w368, "Workspace"=w367, "Tree tag"=w363, "error in (no error)"=w366) -> ("Index out"=w373:T4, "ID"=w372:i32, "Type"=w371:enum16{"I-V", "C-V", "cDLTS", "LDLTS"}, "Canceled"=w370:bool, "error out"=w369:errorcluster)  [unwired: 7 in]
        n129 = case shown="False" w370 {
          tunnel: w369 -> [w400 w494]
          tunnel: w371 -> [w401 _]
          tunnel: w372 -> [w398 _]
          tunnel: w373 -> [w399 w495]
          tunnel: w362 -> [w403 w493]
          tunnel: [w397 w495] -> w378
          tunnel: [w391 w494] -> w377
          tunnel: w381 -> [w394 _]
          tunnel: [w393 w493] -> w380
          tunnel: w367 -> [w390 _]
          tunnel: w375 -> [w389 w492]
          tunnel: [w388 w492] -> w379
          tunnel: w376 -> [w385 _]
          tunnel: w374 -> [w383 _]
          tunnel: w361 -> [w382 _]
          frame False {
            # "Update tree position"
            # "Update tree"
            n130 = case shown="\"I-V\", Default" w401 {
              tunnel: w400 -> [w425 w447 w469 w491]
              tunnel: w399 -> [w421 w443 w465 w487]
              tunnel: w398 -> [w422 w444 w466 w488]
              tunnel: [w419 w441 w463 w485] -> w395
              tunnel: [w418 w440 w462 w484] -> w397
              tunnel: w390 -> [w412 w433 w451 w471]
              tunnel: w389 -> [w410 w435 w453 w474]
              tunnel: [w407 w434 w452 w473] -> w388
              tunnel: [w413 w429 w457 w479] -> w384
              tunnel: w383 -> [w411 w427 w449 w472]
              tunnel: w382 -> [w404 w426 w448 w470]
              frame "I-V", Default {
                n131 = Unbundle By Name(w421) -> ("IV"=w423:T5[])
                n132 = property class="VI"(error in=w425, "FP.State"=T30."Hidden" ("Front Panel Window:State")) -> (error out=w408:errorcluster)  [unwired: 1 in, 1 out]
                n133 = Index Array(array=w423, index=w422) -> (element=w409:T5)
                n134 = call "I-V measurement.vi"("Session properties"=w411, "Workspace"=w412, "Error In"=w408, "myDLTS file path"=w404, "IV measurement"=w409, "Loop data"=w410) -> ("Error Out"=w405:errorcluster, "IV measurement out"=w406:T5, "Loop data out"=w407:T14)  [unwired: 2 in, 1 out]
                n135 = Unbundle By Name(w406) -> ("Name"=w416:string)
                n136 = Replace Array Subset(array=w423, new element=w406, index=w422) -> (w420:T5[])
                n137 = Concatenate Strings("I-V" ("string"), "\\" ("string"), w416) -> (w413:string)
                n138 = property class="VI"(error in=w405, "FP.State"=T30."Standard" ("Front Panel Window:State")) -> (error out=w419:errorcluster)  [unwired: 1 in, 1 out]
                n139 = Bundle By Name(cluster=w421, "IV"=w420) -> (w418:T4)
              }
              frame "C-V" {
                n140 = Unbundle By Name(w443) -> ("CV"=w445:T7[])
                n141 = property class="VI"(error in=w447, "FP.State"=T30."Hidden" ("Front Panel Window:State")) -> (error out=w438:errorcluster)  [unwired: 1 in, 1 out]
                n142 = Index Array(array=w445, index=w444) -> (element=w437:T7)
                n143 = call "C-V measurement.vi"("Session properties"=w427, "Workspace"=w433, "Error In"=w438, "myDLTS file path"=w426, "CV measurement"=w437, "Loop data"=w435) -> ("Error Out"=w436:errorcluster, "CV measurement out"=w428:T7, "Loop data out"=w434:T14)  [unwired: 2 in, 1 out]
                n144 = Unbundle By Name(w428) -> ("Name"=w432:string)
                n145 = property class="VI"(error in=w436, "FP.State"=T30."Standard" ("Front Panel Window:State")) -> (error out=w441:errorcluster)  [unwired: 1 in, 1 out]
                n146 = Replace Array Subset(array=w445, new element=w428, index=w444) -> (w442:T7[])
                n147 = Concatenate Strings("cDLTS" ("string"), "\\" ("string"), w432) -> (w429:string)
                n148 = Bundle By Name(cluster=w443, "CV"=w442) -> (w440:T4)
              }
              frame "cDLTS" {
                n149 = Unbundle By Name(w465) -> ("Conv DLTS"=w467:T11[])
                n150 = Index Array(array=w467, index=w466) -> (element=w450:T11)
                n151 = property class="VI"(error in=w469, "FP.State"=T30."Hidden" ("Front Panel Window:State")) -> (error out=w456:errorcluster)  [unwired: 1 in, 1 out]
                n152 = call "cDLTS measurement.vi"("Session properties"=w449, "Workspace"=w451, "Error In"=w456, "myDLTS file path"=w448, "cDLTS measurement"=w450, "Loop data"=w453) -> ("Error Out"=w455:errorcluster, "cDLTS measurement out"=w454:T11, "Loop data out"=w452:T14)  [unwired: 2 in, 1 out]
                n153 = Unbundle By Name(w454) -> ("Name"=w460:string)
                n154 = Replace Array Subset(array=w467, new element=w454, index=w466) -> (w464:T11[])
                n155 = property class="VI"(error in=w455, "FP.State"=T30."Standard" ("Front Panel Window:State")) -> (error out=w463:errorcluster)  [unwired: 1 in, 1 out]
                n156 = Concatenate Strings("Conventional DLTS" ("string"), "\\" ("string"), w460) -> (w457:string)
                n157 = Bundle By Name(cluster=w465, "Conv DLTS"=w464) -> (w462:T4)
              }
              frame "LDLTS" {
                n158 = Unbundle By Name(w487) -> ("LDLTS"=w489:T9[])
                n159 = Index Array(array=w489, index=w488) -> (element=w476:T9)
                n160 = property class="VI"(error in=w491, "FP.State"=T30."Hidden" ("Front Panel Window:State")) -> (error out=w478:errorcluster)  [unwired: 1 in, 1 out]
                n161 = call "LDLTS measurement.vi"("Session properties"=w472, "Workspace"=w471, "Error In"=w478, "myDLTS file path"=w470, "LDLTS measurement"=w476, "Loop data"=w474) -> ("Error Out"=w477:errorcluster, "LDLTS measurement out"=w475:T9, "Loop data out"=w473:T14)  [unwired: 2 in, 1 out]
                n162 = Unbundle By Name(w475) -> ("Name"=w482:string)
                n163 = Replace Array Subset(array=w489, new element=w475, index=w488) -> (w486:T9[])
                n164 = property class="VI"(error in=w477, "FP.State"=T30."Standard" ("Front Panel Window:State")) -> (error out=w485:errorcluster)  [unwired: 1 in, 1 out]
                n165 = Concatenate Strings("Laplace DLTS" ("string"), "\\" ("string"), w482) -> (w479:string)
                n166 = Bundle By Name(cluster=w487, "LDLTS"=w486) -> (w484:T4)
              }
            }
            n167 = Bundle By Name(cluster=w403, "Saved"=FALSE) -> (w393:cluster{"Saved":bool, "Path":path})
            n168 = Generate User Event(user event=w394, event data cluster=TRUE ("event data"), error in=w395) -> (error out=w387:errorcluster)  [unwired: 1 in, 1 out]
            n169 = Generate User Event(user event=w385, event data cluster=w384, error in=w387) -> (error out=w386:errorcluster)  [unwired: 1 in, 1 out]
            n170 = property on="Save" class="Bool"(error in=w386, "DisabledEnum"=T29."Enabled" ("Disabled")) -> (error out=w391:errorcluster)  [unwired: 1 in, 1 out]
          }
          frame True {
          }
        }
      }
      event "Measurement.View": Value Change; User Event {
        # "Update tree"
        # "Open existing measurement: identyfy type and ID from tree tag, open specific SubVI, set \"Saved\" flag to false and enable \"Save\" button (if applicable)"
        n171 = event-data() -> ()  [unwired: 1 in, 3 out]
        n172 = for {
          tunnel: [w526] -> w496 mode=indexing if=w518
          tunnel: [w525] -> w511 mode=indexing if=w518
          tunnel: "Tree" -> [w524] mode=indexing
          shift-right: [w519] -> _
          shift-left: _ -> [w523]
          i -> [w522]
          # "Measurement index"
          # "Measurement type as ENUM"
          # "Filter measurements of the \nsame type as the first one"
          n173 = String To Path(string=w524) -> (path=w531:path)
          n174 = Path to Array of Strings(0:w531) -> (2:w530:string[])  [unwired: 1 out]
          n175 = Index Array(array=w530, index #1=2 ("index"), index #2=1 ("index")) -> (element #1=w527:string, element #2=w520:string)
          n176 = Equal To 0?(x=w522) -> (x = 0?=w521:bool)
          n177 = Build Array("I-V", "C-V" ("element"), "Conventional DLTS" ("element"), "Laplace DLTS" ("element")) -> (w538:string[])
          n178 = Select(t=w520, s=w521, f=w523) -> (s? t:f=w519:string)
          n179 = Decimal String To Number(string=w527) -> (number=w526:i32)  [unwired: 2 in, 1 out]
          n180 = Equal?(x=w520, y=w519) -> (x = y?=w518:bool)
          n181 = for {
            tunnel: w538 -> [w542] mode=indexing
            tunnel: [w541] -> w537
            tunnel: w520 -> [w539]
            i -> [w541]
            stop <- w540 stop-if-true
            n182 = Equal?(x=w539, y=w542) -> (x = y?=w540:bool)
          }
          n183 = Coerce To Type(0:w537, 1:enum16{"I-V", "C-V", "cDLTS", "LDLTS"}."I-V") -> (2:w525:enum16{"I-V", "C-V", "cDLTS", "LDLTS"})
        }
        n184 = property class="VI"(error in=w517, "FP.State"=T30."Standard" ("Front Panel Window:State")) -> (error out=w510:errorcluster)  [unwired: 1 in, 1 out]
        n185 = Unbundle By Name(w500) -> ("Path"=w499:path)
        n186 = Array Size(array=w496) -> (size(s)=w498:i32)
        n187 = case shown="2, Default" w498 {
          tunnel: w513 -> [w544 w560 w647]
          tunnel: [w544 w559 w647] -> w512
          tunnel: w496 -> [_ w558 w654]
          tunnel: w511 -> [_ w557 w653]
          tunnel: w510 -> [w546 w556 w652]
          tunnel: [w546 w555 w645] -> w507
          tunnel: w505 -> [_ w554 w651]
          tunnel: w504 -> [w543 w553 w637]
          tunnel: [w543 w552 w637] -> w503
          tunnel: [FALSE ("Modified") w551 FALSE ("Modified")] -> w502
          tunnel: w501 -> [_ w550 w638]
          tunnel: w499 -> [_ w549 w650]
          frame 0 {
          }
          frame 1 {
            n188 = Index Array(array=w558) -> (element=w548:i32)  [unwired: 1 in]
            n189 = Index Array(array=w557) -> (element=w547:enum16{"I-V", "C-V", "cDLTS", "LDLTS"})  [unwired: 1 in]
            n190 = case shown="\"LDLTS\"" w547 {
              tunnel: w556 -> [w579 w598 w617 w636]
              tunnel: w560 -> [w575 w594 w613 w632]
              tunnel: w548 -> [w576 w595 w614 w633]
              tunnel: [w573 w592 w611 w630] -> w555
              tunnel: [w572 w591 w610 w629] -> w559
              tunnel: w554 -> [w570 w584 w601 w626]
              tunnel: w553 -> [w568 w585 w605 w625]
              tunnel: [w565 w583 w604 w624] -> w552
              tunnel: [w563 w582 w603 w621] -> w551
              tunnel: w550 -> [w569 w581 w600 w627]
              tunnel: w549 -> [w561 w580 w599 w618]
              frame "I-V", Default {
                n191 = Unbundle By Name(w575) -> ("IV"=w577:T5[])
                n192 = Index Array(array=w577, index=w576) -> (element=w567:T5)
                n193 = property class="VI"(error in=w579, "FP.State"=T30."Hidden" ("Front Panel Window:State")) -> (error out=w566:errorcluster)  [unwired: 1 in, 1 out]
                n194 = call "I-V measurement.vi"("Session properties"=w569, "Workspace"=w570, "Error In"=w566, "myDLTS file path"=w561, "IV measurement"=w567, "Loop data"=w568) -> ("Error Out"=w562:errorcluster, "Modified"=w563:bool, "IV measurement out"=w564:T5, "Loop data out"=w565:T14)  [unwired: 2 in]
                n195 = property class="VI"(error in=w562, "FP.State"=T30."Standard" ("Front Panel Window:State")) -> (error out=w573:errorcluster)  [unwired: 1 in, 1 out]
                n196 = Replace Array Subset(array=w577, new element=w564, index=w576) -> (w574:T5[])
                n197 = Bundle By Name(cluster=w575, "IV"=w574) -> (w572:T4)
              }
              frame "C-V" {
                n198 = Unbundle By Name(w594) -> ("CV"=w596:T7[])
                n199 = Index Array(array=w596, index=w595) -> (element=w588:T7)
                n200 = property class="VI"(error in=w598, "FP.State"=T30."Hidden" ("Front Panel Window:State")) -> (error out=w589:errorcluster)  [unwired: 1 in, 1 out]
                n201 = call "C-V measurement.vi"("Session properties"=w581, "Workspace"=w584, "Error In"=w589, "myDLTS file path"=w580, "CV measurement"=w588, "Loop data"=w585) -> ("Error Out"=w586:errorcluster, "Modified"=w582:bool, "CV measurement out"=w587:T7, "Loop data out"=w583:T14)  [unwired: 2 in]
                n202 = property class="VI"(error in=w586, "FP.State"=T30."Standard" ("Front Panel Window:State")) -> (error out=w592:errorcluster)  [unwired: 1 in, 1 out]
                n203 = Replace Array Subset(array=w596, new element=w587, index=w595) -> (w593:T7[])
                n204 = Bundle By Name(cluster=w594, "CV"=w593) -> (w591:T4)
              }
              frame "cDLTS" {
                n205 = Unbundle By Name(w613) -> ("Conv DLTS"=w615:T11[])
                n206 = Index Array(array=w615, index=w614) -> (element=w607:T11)
                n207 = property class="VI"(error in=w617, "FP.State"=T30."Hidden" ("Front Panel Window:State")) -> (error out=w608:errorcluster)  [unwired: 1 in, 1 out]
                n208 = call "cDLTS measurement.vi"("Session properties"=w600, "Workspace"=w601, "Error In"=w608, "myDLTS file path"=w599, "cDLTS measurement"=w607, "Loop data"=w605) -> ("Error Out"=w602:errorcluster, "Modified"=w603:bool, "cDLTS measurement out"=w606:T11, "Loop data out"=w604:T14)  [unwired: 2 in]
                n209 = Replace Array Subset(array=w615, new element=w606, index=w614) -> (w612:T11[])
                n210 = property class="VI"(error in=w602, "FP.State"=T30."Standard" ("Front Panel Window:State")) -> (error out=w611:errorcluster)  [unwired: 1 in, 1 out]
                n211 = Bundle By Name(cluster=w613, "Conv DLTS"=w612) -> (w610:T4)
              }
              frame "LDLTS" {
                n212 = Unbundle By Name(w632) -> ("LDLTS"=w634:T9[])
                n213 = Index Array(array=w634, index=w633) -> (element=w623:T9)
                n214 = property class="VI"(error in=w636, "FP.State"=T30."Hidden" ("Front Panel Window:State")) -> (error out=w620:errorcluster)  [unwired: 1 in, 1 out]
                n215 = call "LDLTS measurement.vi"("Session properties"=w627, "Workspace"=w626, "Error In"=w620, "myDLTS file path"=w618, "LDLTS measurement"=w623, "Loop data"=w625) -> ("Error Out"=w619:errorcluster, "Modified"=w621:bool, "LDLTS measurement out"=w622:T9, "Loop data out"=w624:T14)  [unwired: 2 in]
                n216 = Replace Array Subset(array=w634, new element=w622, index=w633) -> (w631:T9[])
                n217 = property class="VI"(error in=w619, "FP.State"=T30."Standard" ("Front Panel Window:State")) -> (error out=w630:errorcluster)  [unwired: 1 in, 1 out]
                n218 = Bundle By Name(cluster=w632, "LDLTS"=w631) -> (w629:T4)
              }
            }
          }
          frame 2, Default {
            n219 = Index Array(array=w653) -> (element=w649:enum16{"I-V", "C-V", "cDLTS", "LDLTS"})  [unwired: 1 in]
            n220 = case shown="\"cDLTS\"" w649 {
              tunnel: w652 -> [w669 w684 w699 w714]
              tunnel: w647 -> [w667 w682 w697 w712]
              tunnel: w654 -> [w665 w671 w695 w710]
              tunnel: w651 -> [w656 w674 w690 w701]
              tunnel: w638 -> [w658 w675 w691 w703]
              tunnel: w650 -> [_ _ _ _]
              tunnel: w637 -> [w655 w673 w692 w700]
              tunnel: [w663 w680 w685 w708] -> w640
              tunnel: [w662 w679 w686 w707] -> w641
              tunnel: [w661 w678 w687 w706] -> w642
              tunnel: [w660 w677 w688 w705] -> w643
              tunnel: [w659 w676 w689 w704] -> w644
              frame "LDLTS" {
                n221 = Unbundle By Name(w667) -> ("LDLTS"=w666:T9[])
                n222 = call "Multi Index array.vim"("Indexes"=w665, "Input Array"=w666) -> ("Indexed Subarray"=w657:T9[])
                n223 = property class="VI"(error in=w669, "FP.State"=T30."Hidden" ("Front Panel Window:State")) -> (error out=w664:errorcluster)  [unwired: 1 in, 1 out]
                n224 = call-poly "Parse multiple measurements to display.vi"("Array"=w657, "Session properties"=w658, "Workspace"=w656, "Loop data"=w655, "error in (no error)"=w664) -> ("Plot data"=w659:cluster{"2D data":dbl[], "2D data":dbl[]}[], "Plot names"=w660:string[], "X label"=w661:string, "Y label"=w662:string, "error out"=w663:errorcluster)  [unwired: 6 in]
              }
              frame "I-V" {
                n225 = Unbundle By Name(w682) -> ("IV"=w672:T5[])
                n226 = call "Multi Index array.vim"("Indexes"=w671, "Input Array"=w672) -> ("Indexed Subarray"=w670:T5[])
                n227 = property class="VI"(error in=w684, "FP.State"=T30."Hidden" ("Front Panel Window:State")) -> (error out=w681:errorcluster)  [unwired: 1 in, 1 out]
                n228 = call-poly "Parse multiple measurements to display.vi"("Array"=w670, "Session properties"=w675, "Workspace"=w674, "Loop data"=w673, "error in (no error)"=w681) -> ("Plot data"=w676:cluster{"2D data":dbl[], "2D data":dbl[]}[], "Plot names"=w677:string[], "X label"=w678:string, "Y label"=w679:string, "error out"=w680:errorcluster)  [unwired: 6 in]
              }
              frame "cDLTS" {
                n229 = Unbundle By Name(w697) -> ("Conv DLTS"=w696:T11[])
                n230 = call "Multi Index array.vim"("Indexes"=w695, "Input Array"=w696) -> ("Indexed Subarray"=w693:T11[])
                n231 = property class="VI"(error in=w699, "FP.State"=T30."Hidden" ("Front Panel Window:State")) -> (error out=w694:errorcluster)  [unwired: 1 in, 1 out]
                n232 = call-poly "Parse multiple measurements to display.vi"("Array"=w693, "Session properties"=w691, "Workspace"=w690, "Loop data"=w692, "error in (no error)"=w694) -> ("Plot data"=w689:cluster{"2D data":dbl[], "2D data":dbl[]}[], "Plot names"=w688:string[], "X label"=w687:string, "Y label"=w686:string, "error out"=w685:errorcluster)  [unwired: 6 in]
              }
              frame "C-V" {
                n233 = Unbundle By Name(w712) -> ("CV"=w711:T7[])
                n234 = call "Multi Index array.vim"("Indexes"=w710, "Input Array"=w711) -> ("Indexed Subarray"=w702:T7[])
                n235 = property class="VI"(error in=w714, "FP.State"=T30."Hidden" ("Front Panel Window:State")) -> (error out=w709:errorcluster)  [unwired: 1 in, 1 out]
                n236 = call-poly "Parse multiple measurements to display.vi"("Array"=w702, "Session properties"=w703, "Workspace"=w701, "Loop data"=w700, "error in (no error)"=w709) -> ("Plot data"=w704:cluster{"2D data":dbl[], "2D data":dbl[]}[], "Plot names"=w705:string[], "X label"=w706:string, "Y label"=w707:string, "error out"=w708:errorcluster)  [unwired: 6 in]
              }
            }
            n237 = call "Display multiple measuements.vi"("Plot data"=w644, "Loop data"=w637, "Session properties"=w638, "Plot names"=w643, "X label"=w642, "Y label"=w641, "Error In"=w640) -> ("Error Out"=w639:errorcluster)  [unwired: 8 in]
            n238 = property class="VI"(error in=w639, "FP.State"=T30."Standard" ("Front Panel Window:State")) -> (error out=w645:errorcluster)  [unwired: 1 in, 1 out]
          }
        }
        n239 = case shown="True" w502 {
          tunnel: w500 -> [w716 w725]
          tunnel: [w716 w723] -> w509
          tunnel: [w715 w721] -> w508
          tunnel: w507 -> [w715 w719]
          tunnel: w506 -> [_ w717]
          frame False {
          }
          frame True {
            n240 = Generate User Event(user event=w717, event data cluster=TRUE ("event data"), error in=w719) -> (error out=w718:errorcluster)  [unwired: 1 in, 1 out]
            n241 = Bundle By Name(cluster=w725, "Saved"=FALSE) -> (w723:cluster{"Saved":bool, "Path":path})
            n242 = property on="Save" class="Bool"(error in=w718, "DisabledEnum"=T29."Enabled" ("Disabled")) -> (error out=w721:errorcluster)  [unwired: 1 in, 1 out]
          }
        }
        n243 = property class="VI"(error in=w508, "FP.State"=T30."Standard" ("Front Panel Window:State")) -> (error out=w514:errorcluster)  [unwired: 1 in, 1 out]
      }
      event "Measurement.Delete": Value Change {
        # "Delete measurement: identyfy type and ID from tree tag, open dialog and delete measurement, set \"Saved\" flag to false and enable \"Save\" button (if applicable)"
        n244 = event-data() -> ()  [unwired: 1 in, 1 out]
        n245 = Unbundle By Name(w740) -> ("Saved"=w738:bool)
        n246 = Two Button Dialog(message="Are you sure you want to delete the selected measurements?" ("string"), 2:"Delete" ("T button name (\"OK\")")) -> (T button?=w727:bool)  [unwired: 1 in]
        n247 = property on="Tree" class="Tree (strict)"(error in=w741) -> (error out=w744:errorcluster, "Value"=w728:string[])  [unwired: 1 in, 1 out]
        n248 = case shown="True" w727 {
          tunnel: w744 -> [w747 w760]
          tunnel: w743 -> [w748 w759]
          tunnel: [w748 w758] -> w742
          tunnel: w738 -> [w749 w757]
          tunnel: [w749 w756] -> w734
          tunnel: w732 -> [_ w755]
          tunnel: w730 -> [_ w753]
          tunnel: [w747 w751] -> w729
          tunnel: w728 -> [_ w750]
          frame False {
          }
          frame True {
            n249 = for {
              tunnel: w755 -> [w768]
              shift-right: [w770] -> w752
              shift-left: w760 -> [w774]
              shift-right: [w772] -> w758
              shift-left: w759 -> [w773]
              shift-right: [w769] -> w756
              shift-left: w757 -> [w771]
              tunnel: w750 -> [w761] mode=indexing
              n250 = String To Path(string=w761) -> (path=w767:path)
              n251 = Path to Array of Strings(0:w767) -> (2:w766:string[])  [unwired: 1 out]
              n252 = Index Array(array=w766, index #1=1 ("index"), index #2=2 ("index")) -> (element #1=w763:string, element #2=w762:string)
              n253 = case shown="\"C-V\"" w763 {
                tunnel: w773 -> [w788 w799 w813 w835 w857]
                tunnel: w762 -> [w790 _ w815 w837 w859]
                tunnel: [w786 w799 w811 w833 w855] -> w772
                tunnel: w774 -> [w785 w798 w810 w832 w854]
                tunnel: [w775 w798 w800 w822 w844] -> w770
                tunnel: w771 -> [_ w797 _ _ _]
                tunnel: [FALSE ("Saved") w797 FALSE ("Saved") FALSE ("Saved") FALSE ("Saved")] -> w769
                tunnel: w768 -> [w780 _ w805 w828 w850]
                frame "I-V" {
                  n254 = Unbundle By Name(w788) -> ("IV"=w789:T5[])
                  n255 = Decimal String To Number(string=w790) -> (number=w783:i32)  [unwired: 2 in, 1 out]
                  n256 = Index Array(array=w789, index=w783) -> (element=w791:T5)
                  n257 = Unbundle By Name(w791) -> ("Folder"=w782:path)
                  n258 = Build Path(base path=w780, name or relative path=w782) -> (appended path=w781:path)
                  n259 = call <vilib>:"Check if File or Folder Exists.vi"("error in (no error)"=w785, "path"=w781) -> ("error out"=w778:errorcluster, "file or folder exists?"=w776:bool, "dup path"=w777:path)  [unwired: 7 in]
                  n260 = case shown="True" w776 {
                    tunnel: w777 -> [_ w796]
                    tunnel: w778 -> [w792 w795]
                    tunnel: [w792 w793] -> w775
                    frame False {
                    }
                    frame True {
                      n261 = Delete(path (use dialog)=w796, entire hierarchy (F)=TRUE, error in=w795) -> (error out=w793:errorcluster)  [unwired: 2 in, 2 out]
                    }
                  }
                  n262 = Delete From Array(array=w789, length=1, index=w783) -> (array with subset deleted=w787:T5[])  [unwired: 1 out]
                  n263 = Bundle By Name(cluster=w788, "IV"=w787) -> (w786:T4)
                }
                frame Default {
                }
                frame "C-V" {
                  n264 = Unbundle By Name(w813) -> ("CV"=w814:T7[])
                  n265 = Decimal String To Number(string=w815) -> (number=w808:i32)  [unwired: 2 in, 1 out]
                  n266 = Index Array(array=w814, index=w808) -> (element=w816:T7)
                  n267 = Unbundle By Name(w816) -> ("Folder"=w807:path)
                  n268 = Build Path(base path=w805, name or relative path=w807) -> (appended path=w806:path)
                  n269 = call <vilib>:"Check if File or Folder Exists.vi"("error in (no error)"=w810, "path"=w806) -> ("error out"=w802:errorcluster, "file or folder exists?"=w801:bool, "dup path"=w803:path)  [unwired: 7 in]
                  n270 = Delete From Array(array=w814, length=1, index=w808) -> (array with subset deleted=w812:T7[])  [unwired: 1 out]
                  n271 = case shown="True" w801 {
                    tunnel: [w817 w820] -> w800
                    tunnel: w803 -> [_ w819]
                    tunnel: w802 -> [w817 w818]
                    frame False {
                    }
                    frame True {
                      n272 = Delete(path (use dialog)=w819, entire hierarchy (F)=TRUE, error in=w818) -> (error out=w820:errorcluster)  [unwired: 2 in, 2 out]
                    }
                  }
                  n273 = Bundle By Name(cluster=w813, "CV"=w812) -> (w811:T4)
                }
                frame "Conventional DLTS" {
                  n274 = Unbundle By Name(w835) -> ("Conv DLTS"=w836:T11[])
                  n275 = Decimal String To Number(string=w837) -> (number=w830:i32)  [unwired: 2 in, 1 out]
                  n276 = Index Array(array=w836, index=w830) -> (element=w838:T11)
                  n277 = Unbundle By Name(w838) -> ("Folder"=w829:path)
                  n278 = Build Path(base path=w828, name or relative path=w829) -> (appended path=w827:path)
                  n279 = Delete From Array(array=w836, length=1, index=w830) -> (array with subset deleted=w834:T11[])  [unwired: 1 out]
                  n280 = call <vilib>:"Check if File or Folder Exists.vi"("error in (no error)"=w832, "path"=w827) -> ("error out"=w825:errorcluster, "file or folder exists?"=w823:bool, "dup path"=w824:path)  [unwired: 7 in]
                  n281 = Bundle By Name(cluster=w835, "Conv DLTS"=w834) -> (w833:T4)
                  n282 = case shown="False" w823 {
                    tunnel: w824 -> [_ w843]
                    tunnel: w825 -> [w839 w842]
                    tunnel: [w839 w840] -> w822
                    frame False {
                    }
                    frame True {
                      n283 = Delete(path (use dialog)=w843, entire hierarchy (F)=TRUE, error in=w842) -> (error out=w840:errorcluster)  [unwired: 2 in, 2 out]
                    }
                  }
                }
                frame "Laplace DLTS" {
                  n284 = Unbundle By Name(w857) -> ("LDLTS"=w858:T9[])
                  n285 = Decimal String To Number(string=w859) -> (number=w852:i32)  [unwired: 2 in, 1 out]
                  n286 = Index Array(array=w858, index=w852) -> (element=w860:T9)
                  n287 = Unbundle By Name(w860) -> ("Folder"=w851:path)
                  n288 = Build Path(base path=w850, name or relative path=w851) -> (appended path=w849:path)
                  n289 = Delete From Array(array=w858, length=1, index=w852) -> (array with subset deleted=w856:T9[])  [unwired: 1 out]
                  n290 = call <vilib>:"Check if File or Folder Exists.vi"("error in (no error)"=w854, "path"=w849) -> ("error out"=w845:errorcluster, "file or folder exists?"=w847:bool, "dup path"=w846:path)  [unwired: 7 in]
                  n291 = case shown="True" w847 {
                    tunnel: w846 -> [_ w865]
                    tunnel: w845 -> [w861 w864]
                    tunnel: [w861 w862] -> w844
                    frame False {
                    }
                    frame True {
                      n292 = Delete(path (use dialog)=w865, entire hierarchy (F)=TRUE, error in=w864) -> (error out=w862:errorcluster)  [unwired: 2 in, 2 out]
                    }
                  }
                  n293 = Bundle By Name(cluster=w857, "LDLTS"=w856) -> (w855:T4)
                }
              }
            }
            n294 = Generate User Event(user event=w753, event data cluster=TRUE ("event data"), error in=w752) -> (error out=w751:errorcluster)  [unwired: 1 in, 1 out]
          }
        }
        n295 = Bundle By Name(cluster=w740, "Saved"=w734) -> (w739:cluster{"Saved":bool, "Path":path})
        n296 = Select(t=T29."Disabled and Grayed Out" ("Disabled"), s=w734, f=T29."Enabled") -> (s? t:f=w735:T29)
        n297 = property on="Save" class="Bool"(error in=w729, "DisabledEnum"=w735) -> (error out=w737:errorcluster)  [unwired: 1 in, 1 out]
      }
      event "Measurement.Rename": Value Change {
        # "Rename measurement: identyfy type and ID from tree tag, open rename SubVI dialog, set \"Saved\" flag to false and enable \"Save\" button (if applicable)"
        n298 = event-data() -> ()  [unwired: 1 in, 1 out]
        n299 = property on="Tree" class="Tree (strict)"(error in=w878) -> (error out=w881:errorcluster, "Value"=w867:string[])  [unwired: 1 in, 1 out]
        n300 = Index Array(array=w867) -> (element=w866:string)  [unwired: 1 in]
        n301 = Unbundle By Name(w877) -> ("Saved"=w875:bool)
        n302 = case shown="\"1\", Default" w866 {
          selector: w866 -> [_ w887]
          tunnel: w881 -> [w884 w894]
          tunnel: w880 -> [w886 w893]
          tunnel: [w886 w892] -> w879
          tunnel: w875 -> [w885 w891]
          tunnel: [w884 w890] -> w874
          tunnel: [w885 w889] -> w870
          tunnel: w868 -> [_ w888]
          frame "" {
          }
          frame "1", Default {
            n303 = String To Path(string=w887) -> (path=w900:path)
            n304 = Path to Array of Strings(0:w900) -> (2:w899:string[])  [unwired: 1 out]
            n305 = Index Array(array=w899, index #1=1 ("index"), index #2=2 ("index")) -> (element #1=w896:string, element #2=w895:string)
            n306 = case shown="\"C-V\"" w896 {
              tunnel: w893 -> [w917 w948 w979 w1010 w1027]
              tunnel: w895 -> [w919 w950 w981 w1012 _]
              tunnel: [w915 w946 w977 w1008 w1027] -> w892
              tunnel: w894 -> [w907 w938 w969 w1000 w1026]
              tunnel: [w914 w945 w976 w1007 w1026] -> w890
              tunnel: w891 -> [w913 w944 w975 w1006 w1025]
              tunnel: [w912 w943 w974 w1005 w1025] -> w889
              tunnel: w888 -> [w910 w941 w972 w1003 _]
              frame "I-V" {
                n307 = Unbundle By Name(w917) -> ("IV"=w918:T5[])
                n308 = Decimal String To Number(string=w919) -> (number=w911:i32)  [unwired: 2 in, 1 out]
                n309 = Index Array(array=w918, index=w911) -> (element=w905:T5)
                n310 = Unbundle By Name(w905) -> ("Name"=w909:string, "Comment"=w908:string)
                n311 = call "Measurement renamer.vi"("error in (no error)"=w907, "Comment In"=w908, "Measurement name In"=w909) -> ("error out"=w906:errorcluster, "Canceled"=w902:bool, "Comment Out"=w903:string, "Measurement name Out"=w904:string)  [unwired: 1 in]
                n312 = Bundle By Name(cluster=w905, "Name"=w904, "Comment"=w903) -> (w901:T5)
                n313 = case shown="False" w902 {
                  tunnel: w918 -> [w923 w931]
                  tunnel: [w922 w931] -> w916
                  tunnel: w906 -> [w924 w930]
                  tunnel: [w926 w930] -> w914
                  tunnel: w913 -> [_ w929]
                  tunnel: [FALSE ("Saved") w929] -> w912
                  tunnel: w911 -> [w921 _]
                  tunnel: w910 -> [w925 _]
                  tunnel: w901 -> [w920 _]
                  frame False {
                    n314 = Replace Array Subset(array=w923, new element=w920, index=w921) -> (w922:T5[])
                    n315 = Generate User Event(user event=w925, event data cluster=TRUE ("event data"), error in=w924) -> (error out=w926:errorcluster)  [unwired: 1 in, 1 out]
                  }
                  frame True {
                  }
                }
                n316 = Bundle By Name(cluster=w917, "IV"=w916) -> (w915:T4)
              }
              frame "Laplace DLTS" {
                n317 = Unbundle By Name(w948) -> ("LDLTS"=w949:T9[])
                n318 = Decimal String To Number(string=w950) -> (number=w942:i32)  [unwired: 2 in, 1 out]
                n319 = Index Array(array=w949, index=w942) -> (element=w936:T9)
                n320 = Unbundle By Name(w936) -> ("Name"=w940:string, "Comment"=w939:string)
                n321 = call "Measurement renamer.vi"("error in (no error)"=w938, "Comment In"=w939, "Measurement name In"=w940) -> ("error out"=w937:errorcluster, "Canceled"=w933:bool, "Comment Out"=w934:string, "Measurement name Out"=w935:string)  [unwired: 1 in]
                n322 = Bundle By Name(cluster=w936, "Name"=w935, "Comment"=w934) -> (w932:T9)
                n323 = case shown="False" w933 {
                  tunnel: w949 -> [w954 w962]
                  tunnel: [w953 w962] -> w947
                  tunnel: w937 -> [w955 w961]
                  tunnel: [w957 w961] -> w945
                  tunnel: w944 -> [_ w960]
                  tunnel: [FALSE ("Saved") w960] -> w943
                  tunnel: w942 -> [w952 _]
                  tunnel: w941 -> [w956 _]
                  tunnel: w932 -> [w951 _]
                  frame False {
                    n324 = Replace Array Subset(array=w954, new element=w951, index=w952) -> (w953:T9[])
                    n325 = Generate User Event(user event=w956, event data cluster=TRUE ("event data"), error in=w955) -> (error out=w957:errorcluster)  [unwired: 1 in, 1 out]
                  }
                  frame True {
                  }
                }
                n326 = Bundle By Name(cluster=w948, "LDLTS"=w947) -> (w946:T4)
              }
              frame "Conventional DLTS" {
                n327 = Unbundle By Name(w979) -> ("Conv DLTS"=w980:T11[])
                n328 = Decimal String To Number(string=w981) -> (number=w973:i32)  [unwired: 2 in, 1 out]
                n329 = Index Array(array=w980, index=w973) -> (element=w967:T11)
                n330 = Unbundle By Name(w967) -> ("Name"=w971:string, "Comment"=w970:string)
                n331 = call "Measurement renamer.vi"("error in (no error)"=w969, "Comment In"=w970, "Measurement name In"=w971) -> ("error out"=w968:errorcluster, "Canceled"=w964:bool, "Comment Out"=w965:string, "Measurement name Out"=w966:string)  [unwired: 1 in]
                n332 = Bundle By Name(cluster=w967, "Name"=w966, "Comment"=w965) -> (w963:T11)
                n333 = case shown="False" w964 {
                  tunnel: w980 -> [w985 w993]
                  tunnel: [w984 w993] -> w978
                  tunnel: w968 -> [w986 w992]
                  tunnel: [w988 w992] -> w976
                  tunnel: w975 -> [_ w991]
                  tunnel: [FALSE ("Saved") w991] -> w974
                  tunnel: w973 -> [w983 _]
                  tunnel: w972 -> [w987 _]
                  tunnel: w963 -> [w982 _]
                  frame False {
                    n334 = Replace Array Subset(array=w985, new element=w982, index=w983) -> (w984:T11[])
                    n335 = Generate User Event(user event=w987, event data cluster=TRUE ("event data"), error in=w986) -> (error out=w988:errorcluster)  [unwired: 1 in, 1 out]
                  }
                  frame True {
                  }
                }
                n336 = Bundle By Name(cluster=w979, "Conv DLTS"=w978) -> (w977:T4)
              }
              frame "C-V" {
                n337 = Unbundle By Name(w1010) -> ("CV"=w1011:T7[])
                n338 = Decimal String To Number(string=w1012) -> (number=w1004:i32)  [unwired: 2 in, 1 out]
                n339 = Index Array(array=w1011, index=w1004) -> (element=w998:T7)
                n340 = Unbundle By Name(w998) -> ("Name"=w1002:string, "Comment"=w1001:string)
                n341 = call "Measurement renamer.vi"("error in (no error)"=w1000, "Comment In"=w1001, "Measurement name In"=w1002) -> ("error out"=w999:errorcluster, "Canceled"=w995:bool, "Comment Out"=w996:string, "Measurement name Out"=w997:string)  [unwired: 1 in]
                n342 = Bundle By Name(cluster=w998, "Name"=w997, "Comment"=w996) -> (w994:T7)
                n343 = case shown="False" w995 {
                  tunnel: w1011 -> [w1016 w1024]
                  tunnel: [w1015 w1024] -> w1009
                  tunnel: w999 -> [w1017 w1023]
                  tunnel: [w1019 w1023] -> w1007
                  tunnel: w1006 -> [_ w1022]
                  tunnel: [FALSE ("Saved") w1022] -> w1005
                  tunnel: w1004 -> [w1014 _]
                  tunnel: w1003 -> [w1018 _]
                  tunnel: w994 -> [w1013 _]
                  frame False {
                    n344 = Replace Array Subset(array=w1016, new element=w1013, index=w1014) -> (w1015:T7[])
                    n345 = Generate User Event(user event=w1018, event data cluster=TRUE ("event data"), error in=w1017) -> (error out=w1019:errorcluster)  [unwired: 1 in, 1 out]
                  }
                  frame True {
                  }
                }
                n346 = Bundle By Name(cluster=w1010, "CV"=w1009) -> (w1008:T4)
              }
              frame Default {
              }
            }
          }
        }
        n347 = Bundle By Name(cluster=w877, "Saved"=w870) -> (w876:cluster{"Saved":bool, "Path":path})
        n348 = Select(t=T29."Disabled and Grayed Out" ("Disabled"), s=w870, f=T29."Enabled") -> (s? t:f=w871:T29)
        n349 = property on="Save" class="Bool"(error in=w874, "DisabledEnum"=w871) -> (error out=w873:errorcluster)  [unwired: 1 in, 1 out]
      }
      event "Session.Information": Value Change {
        # "Display session info"
        n350 = event-data() -> ()  [unwired: 1 in, 1 out]
        n351 = call "Session info dialog.vi"("Error In"=w1037, "Session properties in"=w1035) -> ("Error Out"=w1036:errorcluster, "Session properties out"=w1034:T13)  [unwired: 8 in]
        n352 = Unbundle By Name(w1030) -> ("Saved"=w1032:bool)
        n353 = Equal?(x=w1035, y=w1034) -> (x = y?=w1033:bool)
        n354 = Select(t=w1032, s=w1033, f=FALSE) -> (s? t:f=w1029:bool)
        n355 = Bundle By Name(cluster=w1030, "Saved"=w1029) -> (w1028:cluster{"Saved":bool, "Path":path})
      }
      event "Session.Merge": Value Change {
        n356 = event-data() -> ()  [unwired: 1 in, 6 out]
        n357 = call "Session merge.vi"("Loop Data"=w1050, "Error In"=w1052, "Workspace"=w1051, "Index In"=w1048, "Session properties in"=w1049) -> ("Error Out"=w1044:errorcluster, "Imported measurements count"=w1045:i32, "Index Out"=w1046:T4, "Session properties out"=w1047:T13)  [unwired: 3 in]
        n358 = case shown="0" w1045 {
          tunnel: w1044 -> [w1054 w1058]
          tunnel: [w1054 w1059] -> w1043
          tunnel: w1042 -> [_ w1061]
          tunnel: w1041 -> [w1053 w1057]
          tunnel: [w1053 w1056] -> w1040
          frame 0 {
            # "Nothing was imported"
          }
          frame 1, Default {
            # "Reload tree"
            # "At least 1 measurement was imported"
            n359 = Bundle By Name(cluster=w1057, "Saved"=FALSE) -> (w1056:cluster{"Saved":bool, "Path":path})
            n360 = Generate User Event(user event=w1061, event data cluster=TRUE ("event data"), error in=w1058) -> (error out=w1059:errorcluster)  [unwired: 1 in, 1 out]
          }
        }
      }
      event "Session.Save": Value Change; User Event {
        n361 = event-data() -> ()  [unwired: 1 in, 1 out]
        n362 = Unbundle By Name(w1071) -> ("Path"=w1073:path)
        n363 = Bundle By Name(cluster=w1071, "Saved"=TRUE) -> (w1070:cluster{"Saved":bool, "Path":path})
        n364 = call "Save myDLTS file (SubVI).vi"("Loop data in"=w1068, "Index"=w1069, "Session properties"=w1067, "Workspace path"=w1074, "File"=w1073, "Error In"=w1075) -> ("Loop data out"=w1066:T14, "Session properties out"=w1065:T13, "Error  out"=w1064:errorcluster)  [unwired: 5 in, 2 out]
        n365 = property on="Save" class="Bool"(error in=w1064, "DisabledEnum"=T29."Disabled and Grayed Out" ("Disabled")) -> (error out=w1063:errorcluster)  [unwired: 1 in, 1 out]
      }
      event User Event {
        # "Create top level node"
        # "Clear tree"
        # "Render tree list"
        n366 = event-data() -> ()  [unwired: 1 in, 1 out]
        n367 = Unbundle By Name(w1096) -> ("Session name"=w1081:string, "Created"=w1088:timestamp, "Comment"=w1087:string)
        n368 = invoke on="Tree" class="Tree (strict)" method="Edit Tree Items.Delete"(error in=w1102) -> (error out=w1101:errorcluster)  [unwired: 4 in, 4 out]
        n369 = Format Date/Time String(seconds (now)=w1088) -> (date/time string=w1089:string)  [unwired: 2 in]
        n370 = Unbundle By Name(w1097) -> ("IV"=w1079:T5[], "CV"=w1080:T7[], "LDLTS"=w1085:T9[], "Conv DLTS"=w1095:T11[])
        n371 = Build Array(w1089, w1087) -> (w1086:string[])
        n372 = invoke on="Tree" class="Tree (strict)" method="Edit Tree Items.Add Item"(error in=w1101, "Left Cell"=w1081, "Child Text"=w1086, "Child Tag"=w1081) -> (error out=w1100:errorcluster)  [unwired: 5 in, 8 out]
        n373 = Array Size(array=w1079) -> (size(s)=w1091:i32)
        n374 = Array Size(array=w1080) -> (size(s)=w1090:i32)
        n375 = Array Size(array=w1085) -> (size(s)=w1092:i32)
        n376 = Array Size(array=w1095) -> (size(s)=w1094:i32)
        n377 = Greater Than 0?(x=w1091) -> (x > 0?=w1082:bool)
        n378 = Greater Than 0?(x=w1090) -> (x > 0?=w1083:bool)
        n379 = Greater Than 0?(x=w1092) -> (x > 0?=w1084:bool)
        n380 = Greater Than 0?(x=w1094) -> (x > 0?=w1093:bool)
        n381 = stacked-sequence {
          seq-local: [w1103 _ _ _] -> [_ w1141 _ _]
          seq-local: [_ w1138 _ _] -> [_ _ w1173 _]
          seq-local: [_ _ w1172 _] -> [_ _ _ w1206]
          tunnel: w1100 -> [w1110 _ _ _]
          tunnel: w1081 -> [w1106 w1137 w1171 w1205]
          tunnel: w1095 -> [w1105 _ _ _]
          tunnel: w1093 -> [w1104 _ _ _]
          tunnel: w1085 -> [_ w1140 _ _]
          tunnel: w1084 -> [_ w1139 _ _]
          tunnel: w1083 -> [_ _ w1176 _]
          tunnel: w1080 -> [_ _ w1174 _]
          tunnel: w1082 -> [_ _ _ w1210]
          tunnel: w1079 -> [_ _ _ w1208]
          tunnel: [_ _ _ w1207] -> w1078
          frame #0 {
            w1108 = "Conventional DLTS" ("string")
            n382 = Concatenate Strings(w1106, "\\" ("string"), w1108) -> (w1107:string)
            n383 = case shown="True" w1104 {
              tunnel: w1110 -> [w1111 w1120]
              tunnel: w1108 -> [_ w1119]
              tunnel: w1107 -> [_ w1112]
              tunnel: [w1111 w1118] -> w1103
              tunnel: w1106 -> [_ w1117]
              tunnel: w1105 -> [_ w1116]
              frame False {
              }
              frame True {
                # "Create DLTS section"
                n384 = invoke on="Tree" class="Tree (strict)" method="Edit Tree Items.Add Item"(error in=w1120, "Parent Tag"=w1117, "Left Cell"=w1119, "Child Tag"=w1112) -> (error out=w1115:errorcluster)  [unwired: 5 in, 8 out]
                n385 = property on="Tree" class="Tree (strict)"(error in=w1115, "Active Item Tag"=w1112, "Glyph"=15 ("Active Item:Symbol Index")) -> (error out=w1114:errorcluster)  [unwired: 1 in, 1 out]
                n386 = for {
                  tunnel: w1114 -> [w1136]
                  tunnel: w1116 -> [w1135] mode=indexing
                  tunnel: w1112 -> [w1129]
                  tunnel: [w1122] -> w1118
                  i -> [w1127]
                  # "Create measurement section"
                  n387 = Unbundle By Name(w1135) -> ("Name"=w1128:string, "Time"=w1134:timestamp, "Comment"=w1132:string)
                  n388 = Number To Decimal String(number=w1127) -> (decimal integer string=w1126:string)  [unwired: 1 in]
                  n389 = Format Date/Time String(seconds (now)=w1134) -> (date/time string=w1133:string)  [unwired: 2 in]
                  n390 = Concatenate Strings(w1129, "\\" ("string"), w1126) -> (w1121:string)
                  n391 = Build Array(w1133, w1132) -> (w1131:string[])
                  n392 = invoke on="Tree" class="Tree (strict)" method="Edit Tree Items.Add Item"(error in=w1136, "Parent Tag"=w1129, "Left Cell"=w1128, "Child Text"=w1131, "Child Tag"=w1121, "Child Only?"=TRUE) -> (error out=w1123:errorcluster)  [unwired: 3 in, 8 out]
                  n393 = property on="Tree" class="Tree (strict)"(error in=w1123, "Active Item Tag"=w1121, "Glyph"=13 ("Active Item:Symbol Index")) -> (error out=w1122:errorcluster)  [unwired: 1 in, 1 out]
                }
              }
            }
          }
          frame #1 {
            w1143 = "Laplace DLTS" ("string")
            n394 = Concatenate Strings(w1137, "\\" ("string"), w1143) -> (w1142:string)
            n395 = case shown="True" w1139 {
              tunnel: w1142 -> [_ w1148]
              tunnel: w1141 -> [w1145 w1154]
              tunnel: w1143 -> [_ w1153]
              tunnel: w1140 -> [_ w1152]
              tunnel: w1137 -> [_ w1151]
              tunnel: [w1145 w1146] -> w1138
              frame False {
              }
              frame True {
                # "Create LDLTS section"
                n396 = invoke on="Tree" class="Tree (strict)" method="Edit Tree Items.Add Item"(error in=w1154, "Parent Tag"=w1151, "Left Cell"=w1153, "Child Tag"=w1148) -> (error out=w1150:errorcluster)  [unwired: 5 in, 8 out]
                n397 = property on="Tree" class="Tree (strict)"(error in=w1150, "Active Item Tag"=w1148, "Glyph"=15 ("Active Item:Symbol Index")) -> (error out=w1149:errorcluster)  [unwired: 1 in, 1 out]
                n398 = for {
                  tunnel: w1149 -> [w1170]
                  tunnel: w1152 -> [w1169] mode=indexing
                  tunnel: w1148 -> [w1163]
                  tunnel: [w1157] -> w1146
                  i -> [w1161]
                  # "Create measurement section"
                  n399 = Unbundle By Name(w1169) -> ("Name"=w1162:string, "Time"=w1168:timestamp, "Comment"=w1166:string)
                  n400 = Number To Decimal String(number=w1161) -> (decimal integer string=w1160:string)  [unwired: 1 in]
                  n401 = Format Date/Time String(seconds (now)=w1168) -> (date/time string=w1167:string)  [unwired: 2 in]
                  n402 = Concatenate Strings(w1163, "\\" ("string"), w1160) -> (w1156:string)
                  n403 = Build Array(w1167, w1166) -> (w1165:string[])
                  n404 = invoke on="Tree" class="Tree (strict)" method="Edit Tree Items.Add Item"(error in=w1170, "Parent Tag"=w1163, "Left Cell"=w1162, "Child Text"=w1165, "Child Tag"=w1156, "Child Only?"=TRUE) -> (error out=w1158:errorcluster)  [unwired: 3 in, 8 out]
                  n405 = property on="Tree" class="Tree (strict)"(error in=w1158, "Active Item Tag"=w1156, "Glyph"=13 ("Active Item:Symbol Index")) -> (error out=w1157:errorcluster)  [unwired: 1 in, 1 out]
                }
              }
            }
          }
          frame #2 {
            w1177 = "C-V" ("string")
            n406 = Concatenate Strings(w1171, "\\" ("string"), w1177) -> (w1175:string)
            n407 = case shown="True" w1176 {
              tunnel: w1175 -> [_ w1181]
              tunnel: w1173 -> [w1179 w1188]
              tunnel: w1177 -> [_ w1187]
              tunnel: w1174 -> [_ w1186]
              tunnel: [w1179 w1185] -> w1172
              tunnel: w1171 -> [_ w1184]
              frame False {
              }
              frame True {
                # "Create C-V section"
                n408 = invoke on="Tree" class="Tree (strict)" method="Edit Tree Items.Add Item"(error in=w1188, "Parent Tag"=w1184, "Left Cell"=w1187, "Child Tag"=w1181) -> (error out=w1182:errorcluster)  [unwired: 5 in, 8 out]
                n409 = property on="Tree" class="Tree (strict)"(error in=w1182, "Active Item Tag"=w1181, "Glyph"=15 ("Active Item:Symbol Index")) -> (error out=w1183:errorcluster)  [unwired: 1 in, 1 out]
                n410 = for {
                  tunnel: w1183 -> [w1204]
                  tunnel: w1186 -> [w1203] mode=indexing
                  tunnel: w1181 -> [w1197]
                  tunnel: [w1192] -> w1185
                  i -> [w1195]
                  # "Create measurement section"
                  n411 = Unbundle By Name(w1203) -> ("Name"=w1196:string, "Time"=w1202:timestamp, "Comment"=w1200:string)
                  n412 = Number To Decimal String(number=w1195) -> (decimal integer string=w1194:string)  [unwired: 1 in]
                  n413 = Format Date/Time String(seconds (now)=w1202) -> (date/time string=w1201:string)  [unwired: 2 in]
                  n414 = Concatenate Strings(w1197, "\\" ("string"), w1194) -> (w1190:string)
                  n415 = Build Array(w1201, w1200) -> (w1199:string[])
                  n416 = invoke on="Tree" class="Tree (strict)" method="Edit Tree Items.Add Item"(error in=w1204, "Parent Tag"=w1197, "Left Cell"=w1196, "Child Text"=w1199, "Child Tag"=w1190, "Child Only?"=TRUE) -> (error out=w1191:errorcluster)  [unwired: 3 in, 8 out]
                  n417 = property on="Tree" class="Tree (strict)"(error in=w1191, "Active Item Tag"=w1190, "Glyph"=13 ("Active Item:Symbol Index")) -> (error out=w1192:errorcluster)  [unwired: 1 in, 1 out]
                }
              }
            }
          }
          frame #3 {
            w1211 = "I-V" ("string")
            n418 = Concatenate Strings(w1205, "\\" ("string"), w1211) -> (w1209:string)
            n419 = case shown="True" w1210 {
              tunnel: w1209 -> [_ w1214]
              tunnel: w1206 -> [w1213 w1222]
              tunnel: w1205 -> [_ w1221]
              tunnel: w1211 -> [_ w1220]
              tunnel: w1208 -> [_ w1219]
              tunnel: [w1213 w1218] -> w1207
              frame False {
              }
              frame True {
                # "Create I-V section"
                n420 = invoke on="Tree" class="Tree (strict)" method="Edit Tree Items.Add Item"(error in=w1222, "Parent Tag"=w1221, "Left Cell"=w1220, "Child Tag"=w1214) -> (error out=w1217:errorcluster)  [unwired: 5 in, 8 out]
                n421 = property on="Tree" class="Tree (strict)"(error in=w1217, "Active Item Tag"=w1214, "Glyph"=15 ("Active Item:Symbol Index")) -> (error out=w1216:errorcluster)  [unwired: 1 in, 1 out]
                n422 = for {
                  tunnel: w1216 -> [w1238]
                  tunnel: w1219 -> [w1237] mode=indexing
                  tunnel: w1214 -> [w1231]
                  tunnel: [w1225] -> w1218
                  i -> [w1228]
                  # "Create measurement section"
                  n423 = Unbundle By Name(w1237) -> ("Name"=w1230:string, "Time"=w1236:timestamp, "Comment"=w1234:string)
                  n424 = Number To Decimal String(number=w1228) -> (decimal integer string=w1227:string)  [unwired: 1 in]
                  n425 = Format Date/Time String(seconds (now)=w1236) -> (date/time string=w1235:string)  [unwired: 2 in]
                  n426 = Concatenate Strings(w1231, "\\" ("string"), w1227) -> (w1223:string)
                  n427 = Build Array(w1235, w1234) -> (w1233:string[])
                  n428 = invoke on="Tree" class="Tree (strict)" method="Edit Tree Items.Add Item"(error in=w1238, "Parent Tag"=w1231, "Left Cell"=w1230, "Child Text"=w1233, "Child Tag"=w1223, "Child Only?"=TRUE) -> (error out=w1226:errorcluster)  [unwired: 3 in, 8 out]
                  n429 = property on="Tree" class="Tree (strict)"(error in=w1226, "Active Item Tag"=w1223, "Glyph"=13 ("Active Item:Symbol Index")) -> (error out=w1225:errorcluster)  [unwired: 1 in, 1 out]
                }
              }
            }
          }
        }
        n430 = property on="Tree" class="Tree (strict)"(error in=w1078, "Val(Sgnl)"=string[] [] ("Value (Signaling)")) -> (error out=w1077:errorcluster)  [unwired: 1 in, 1 out]
      }
      event "Tree": Double Click {
        n431 = event-data() -> ("Tag"=w1243:string)  [unwired: 1 in]
        n432 = String To Path(string=w1243) -> (path=w1244:path)
        n433 = Path to Array of Strings(0:w1244) -> (2:w1242:string[])  [unwired: 1 out]
        n434 = Array Size(array=w1242) -> (size(s)=w1241:i32)
        n435 = Greater Or Equal?(x=w1241, y=3) -> (x >= y?=w1240:bool)
        n436 = case shown="True" w1240 {
          tunnel: w1247 -> [w1252 w1256]
          tunnel: [w1252 w1255] -> w1246
          tunnel: w1245 -> [_ w1253]
          frame False {
          }
          frame True {
            n437 = Generate User Event(user event=w1253, event data cluster=TRUE ("event data"), error in=w1256) -> (error out=w1255:errorcluster)  [unwired: 1 in, 1 out]
          }
        }
      }
      event "Tree": Value Change {
        # "Enable buttons if tree points to a measurement (disable otherwise)"
        n438 = event-data() -> ("NewVal"=w1260:string[])  [unwired: 1 in]
        n439 = Array Size(array=w1260) -> (size(s)=w1259:i32)
        n440 = case shown="0, Default" w1259 {
          tunnel: [T29."Disabled and Grayed Out" ("Disabled") T29."Enabled" ("Disabled") T29."Enabled" ("Disabled")] -> w1257
          tunnel: [T29."Disabled and Grayed Out" ("Disabled") T29."Enabled" ("Disabled") T29."Disabled and Grayed Out" ("Disabled")] -> w1258
          tunnel: [T29."Disabled and Grayed Out" ("Disabled") T29."Disabled and Grayed Out" ("Disabled") T29."Enabled" ("Disabled")] -> _
          frame 0, Default {
          }
          frame 1 {
          }
          frame 2.. {
          }
        }
        n441 = property on="Export" class="Bool"(error in=w1265, "DisabledEnum"=w1257) -> (error out=w1264:errorcluster)  [unwired: 1 in, 1 out]
        n442 = property on="View" class="Bool"(error in=w1264, "DisabledEnum"=w1257) -> (error out=w1270:errorcluster)  [unwired: 1 in, 1 out]
        n443 = property on="Delete" class="Bool"(error in=w1270, "DisabledEnum"=w1257) -> (error out=w1263:errorcluster)  [unwired: 1 in, 1 out]
        n444 = property on="Rename" class="Bool"(error in=w1263, "DisabledEnum"=w1258) -> (error out=w1262:errorcluster)  [unwired: 1 in, 1 out]
        n445 = property on="Copy" class="Bool"(error in=w1262, "DisabledEnum"=w1258) -> (error out=w1261:errorcluster)  [unwired: 1 in, 1 out]
      }
      event User Event {
        # "Highlight given measurement"
        n446 = event-data() -> ("Change tree position"=w1285:string)  [unwired: 1 in]
        n447 = case shown="Default" w1285 {
          selector: w1285 -> [_ w1297]
          tunnel: w1284 -> [_ w1298]
          tunnel: [w1291 w1292] -> w1281
          tunnel: w1283 -> [w1290 w1293]
          tunnel: [w1289 w1293] -> w1282
          frame "" {
            n448 = property on="Tree" class="Tree (strict)"(error in=w1290) -> (error out=w1289:errorcluster, "Value"=w1291:string[])  [unwired: 1 in, 1 out]
          }
          frame Default {
            n449 = Unbundle By Name(w1298) -> ("Session name"=w1296:string)
            n450 = Concatenate Strings(w1296, "\\" ("string"), w1297) -> (w1294:string)
            n451 = Build Array(w1294) -> (w1292:string[])
          }
        }
        n452 = property on="Tree" class="Tree (strict)"(error in=w1282, "Val(Sgnl)"=w1281) -> (error out=w1280:errorcluster)  [unwired: 1 in, 1 out]
      }
      event "Measurement.Export": Value Change {
        # "Export data"
        n453 = event-data() -> ("NewVal"=w1299:bool)  [unwired: 1 in]
        n454 = case shown="True" w1299 {
          tunnel: w1306 -> [w1307 w1328]
          tunnel: w1304 -> [_ w1327]
          tunnel: w1303 -> [_ w1326]
          tunnel: [w1307 w1325] -> w1302
          tunnel: w1301 -> [_ w1324]
          tunnel: w1300 -> [_ w1323]
          frame False {
          }
          frame True {
            # "Only execute when button changes value to true"
            # "Export type dialog"
            # "Posible export types"
            n455 = property on="Tree" class="Tree (strict)"(error in=w1328) -> (error out=w1319:errorcluster, "Value"=w1316:string[])  [unwired: 1 in, 1 out]
            n456 = for {
              tunnel: [w1336] -> w1311 mode=indexing if=w1329
              tunnel: [w1335] -> w1315 mode=indexing if=w1329
              tunnel: w1316 -> [w1330] mode=indexing
              shift-right: [w1331] -> w1314
              shift-left: _ -> [w1332]
              tunnel: [w1330] -> _ mode=indexing if=w1329
              i -> [w1334]
              # "Filter tags to match the type of the first measutement"
              n457 = String To Path(string=w1330) -> (path=w1339:path)
              n458 = Equal To 0?(x=w1334) -> (x = 0?=w1333:bool)
              n459 = Path to Array of Strings(0:w1339) -> (2:w1340:string[])  [unwired: 1 out]
              n460 = Select(t=w1330, s=w1333, f=w1332) -> (s? t:f=w1331:string)
              n461 = Index Array(array=w1340, index #1=2 ("index"), index #2=1 ("index")) -> (element #1=w1341:string, element #2=w1335:string)
              n462 = Equal?(x=w1330, y=w1331) -> (x = y?=w1329:bool)
              n463 = Decimal String To Number(string=w1341) -> (number=w1336:i32)  [unwired: 2 in, 1 out]
            }
            n464 = Unbundle By Name(w1324) -> ("Settings.Other.Enable OriginLab"=w1322:bool)
            n465 = Array Size(array=w1311) -> (size(s)=w1310:i32)
            n466 = Equal?(x=1, y=w1310) -> (x = y?=w1308:bool)
            n467 = Equal?(x="Laplace DLTS", y=w1314) -> (x = y?=w1318:bool)
            n468 = Bundle By Name(cluster=T31 {"Clipboard"=FALSE, "dat"=TRUE, "iso"=FALSE, "Origin"=FALSE, "Excel"=FALSE} ("Available options"), "Origin"=w1322, "iso"=w1318, "Clipboard"=w1308) -> (w1312:T31)
            n469 = call "Export dialog.vi"("error in (no error)"=w1319, "Available options"=w1312) -> ("error out"=w1321:errorcluster, "Option"=w1320:T36)  [unwired: 7 in, 1 out]
            n470 = case shown="\"Clipboard\"" w1320 {
              tunnel: w1327 -> [_ w1344 w1385 w1394]
              tunnel: w1326 -> [_ w1345 w1384 w1393]
              tunnel: [w1342 w1343 w1381 w1392] -> w1325
              tunnel: w1321 -> [w1342 w1348 w1380 w1388]
              tunnel: w1323 -> [_ _ _ w1391]
              tunnel: w1311 -> [_ w1346 _ w1390]
              tunnel: w1315 -> [_ w1347 _ w1389]
              tunnel: w1316 -> [_ _ w1382 _]
              frame "Canceled", Default {
                # "Export was canceled"
              }
              frame "Clipboard" {
                # "Export only one at a time"
                n471 = Index Array(array=w1346) -> (element=w1350:i32)  [unwired: 1 in]
                n472 = Index Array(array=w1347) -> (element=w1349:string)  [unwired: 1 in]
                n473 = case shown="\"C-V\"" w1349 {
                  tunnel: w1350 -> [_ w1357 w1364 w1371 w1378]
                  tunnel: w1344 -> [_ w1356 w1363 w1370 w1377]
                  tunnel: [w1351 w1352 w1359 w1366 w1373] -> w1343
                  tunnel: w1348 -> [w1351 w1355 w1360 w1369 w1376]
                  tunnel: w1345 -> [_ w1354 w1361 w1368 w1375]
                  frame Default {
                  }
                  frame "Conventional DLTS" {
                    n474 = Unbundle By Name(w1356) -> ("Conv DLTS"=w1358:T11[])
                    n475 = Index Array(array=w1358, index=w1357) -> (element=w1353:T11)
                    n476 = call-poly "Export single clipboard - cluster.vi"("Error In"=w1355, "Workspace"=w1354, "cDLTS measurement"=w1353) -> ("Error Out"=w1352:errorcluster)  [unwired: 5 in]
                  }
                  frame "C-V" {
                    n477 = Unbundle By Name(w1363) -> ("CV"=w1365:T7[])
                    n478 = Index Array(array=w1365, index=w1364) -> (element=w1362:T7)
                    n479 = call-poly "Export single clipboard - cluster.vi"("Error In"=w1360, "Workspace"=w1361, "CV measurement"=w1362) -> ("Error Out"=w1359:errorcluster)  [unwired: 5 in]
                  }
                  frame "Laplace DLTS" {
                    n480 = Unbundle By Name(w1370) -> ("LDLTS"=w1372:T9[])
                    n481 = Index Array(array=w1372, index=w1371) -> (element=w1367:T9)
                    n482 = call-poly "Export single clipboard - cluster.vi"("Error In"=w1369, "Workspace"=w1368, "LDLTS measurement"=w1367) -> ("Error Out"=w1366:errorcluster)  [unwired: 5 in]
                  }
                  frame "I-V" {
                    n483 = Unbundle By Name(w1377) -> ("IV"=w1379:T5[])
                    n484 = Index Array(array=w1379, index=w1378) -> (element=w1374:T5)
                    n485 = call-poly "Export single clipboard - cluster.vi"("Error In"=w1376, "Workspace"=w1375, "IV measurement"=w1374) -> ("Error Out"=w1373:errorcluster)  [unwired: 5 in]
                  }
                }
              }
              frame "Dat" {
                # "Export to text based .dat file"
                n486 = local read "Actual file"() -> (w1383:path)
                n487 = call "Export multiple dat - tag.vi"(".myDLTS file path"=w1383, "Error In"=w1380, "Workspace"=w1384, "Index"=w1385, "Measurement tags"=w1382) -> ("Error Out"=w1381:errorcluster)  [unwired: 3 in]
              }
              frame "Origin" {
                # "Export only one at a time"
                # "Export to Origin Lab\nDEPRECATED"
                n488 = Index Array(array=w1390) -> (element=w1386:i32)  [unwired: 1 in]
                n489 = Index Array(array=w1389) -> (element=w1387:string)  [unwired: 1 in]
                n490 = case shown="\"Conventional DLTS\"" w1387 {
                  tunnel: w1386 -> [_ w1402 w1410 w1418 w1426]
                  tunnel: w1394 -> [_ w1401 w1409 w1417 w1425]
                  tunnel: [w1395 w1399 w1407 w1413 w1421] -> w1392
                  tunnel: w1388 -> [w1395 w1400 w1408 w1414 w1422]
                  tunnel: w1393 -> [_ w1396 w1405 w1415 w1420]
                  tunnel: w1391 -> [_ w1398 w1404 w1412 w1424]
                  frame Default {
                  }
                  frame "I-V" {
                    n491 = Unbundle By Name(w1401) -> ("IV"=w1403:T5[])
                    n492 = Index Array(array=w1403, index=w1402) -> (element=w1397:T5)
                    n493 = call-poly "Export Origin.vi"("Error In"=w1400, "Workspace"=w1396, "Session properties"=w1398, "IV measurement"=w1397) -> ("Error Out"=w1399:errorcluster)  [unwired: 7 in]
                  }
                  frame "C-V" {
                    n494 = Unbundle By Name(w1409) -> ("CV"=w1411:T7[])
                    n495 = Index Array(array=w1411, index=w1410) -> (element=w1406:T7)
                    n496 = call-poly "Export Origin.vi"("Error In"=w1408, "Workspace"=w1405, "Session properties"=w1404, "CV measurement"=w1406) -> ("Error Out"=w1407:errorcluster)  [unwired: 7 in]
                  }
                  frame "Conventional DLTS" {
                    n497 = Unbundle By Name(w1417) -> ("Conv DLTS"=w1419:T11[])
                    n498 = Index Array(array=w1419, index=w1418) -> (element=w1416:T11)
                    n499 = call-poly "Export Origin.vi"("Error In"=w1414, "Workspace"=w1415, "Session properties"=w1412, "cDLTS measurement"=w1416) -> ("Error Out"=w1413:errorcluster)  [unwired: 7 in]
                  }
                  frame "Laplace DLTS" {
                    n500 = Unbundle By Name(w1425) -> ("LDLTS"=w1427:T9[])
                    n501 = Index Array(array=w1427, index=w1426) -> (element=w1423:T9)
                    n502 = call-poly "Export Origin.vi"("Error In"=w1422, "Workspace"=w1420, "Session properties"=w1424, "LDLTS measurement"=w1423) -> ("Error Out"=w1421:errorcluster)  [unwired: 7 in]
                  }
                }
              }
            }
          }
        }
      }
      event "Devices.MFIA.MFIA Connect", "Devices.Source meter.SM Connect", "Devices.Temperature controler.TC Connect": Value Change {
        # "Connect or disconnect device"
        n503 = event-data() -> ("CtlRef"=w1435:refnum<vi>, "NewVal"=w1434:bool)  [unwired: 1 in]
        n504 = control-ref of="MFIA Connect"() -> (w1439:refnum<vi>)
        n505 = control-ref of="SM Connect"() -> (w1438:refnum<vi>)
        n506 = control-ref of="TC Connect"() -> (w1437:refnum<vi>)
        n507 = Build Array(w1439, w1438, w1437) -> (w1436:refnum<vi>[])
        n508 = Search 1D Array(1D array=w1436, element=w1435) -> (index of element=w1433:i32)  [unwired: 1 in]
        n509 = case shown="2" w1433 {
          tunnel: [T32 {"MFIA"=FALSE, "Temperature controller"=FALSE, "Source meter"=FALSE} ("Devices") T32 {"MFIA"=TRUE, "Temperature controller"=FALSE, "Source meter"=FALSE} ("Devices") T32 {"MFIA"=FALSE, "Temperature controller"=FALSE, "Source meter"=TRUE} ("Devices") T32 {"MFIA"=FALSE, "Temperature controller"=TRUE, "Source meter"=FALSE} ("Devices")] -> w1432
          frame -1, Default {
          }
          frame 0 {
          }
          frame 1 {
          }
          frame 2 {
          }
        }
        n510 = case shown="True" w1434 {
          tunnel: w1432 -> [w1451 w1454]
          tunnel: w1431 -> [w1450 w1456]
          tunnel: w1429 -> [w1449 w1455]
          tunnel: [w1448 w1453] -> w1430
          tunnel: [w1447 w1452] -> w1428
          frame False {
            n511 = call "Disconnect devices (SubVI).vi"("error in (no error)"=w1449, "Devices"=w1451, "Loop data"=w1450) -> ("Error Out"=w1447:errorcluster, "Loop data out"=w1448:T14)  [unwired: 7 in]
          }
          frame True {
            n512 = call "Connect devices (SubIV).vi"("Error In"=w1455, "Devices"=w1454, "Loop data in"=w1456) -> ("Error Out"=w1452:errorcluster, "Loop data out"=w1453:T14)  [unwired: 6 in, 1 out]
          }
        }
      }
      event "Devices.Temperature controler.Setpoint": Value Change {
        # "Set temperature setpoint"
        n513 = event-data() -> ("NewVal"=w1461:dbl[unit])  [unwired: 1 in]
        n514 = Unbundle By Name(w1458) -> ("Temp handle"=w1457:T16)
        n515 = call "Temp ctrl - Setpoint.vi"("Error In"=w1460, "Setpoint"=w1461, "Temp handle"=w1457) -> ("Error Out"=w1459:errorcluster)  [unwired: 8 in]
      }
      event "Devices.MFIA.Power": Value Change {
        # "Shut down MFIA"
        n516 = event-data() -> ()  [unwired: 1 in, 1 out]
        n517 = call "Disconnect devices (SubVI).vi"("error in (no error)"=w1470, "Force turn off MFIA"=TRUE, "Devices"=T32 {"MFIA"=TRUE, "Temperature controller"=FALSE, "Source meter"=FALSE}, "Loop data"=w1468) -> ("Error Out"=w1469:errorcluster, "Loop data out"=w1467:T14)  [unwired: 6 in]
      }
    }
    n518 = call <vilib>:"General Error Handler.vi"("type of dialog (OK msg:1)"=w74, "error in (no error)"=w75) -> ("code out"=w72:i32, "error out"=w73:errorcluster)  [unwired: 9 in, 3 out]
    n519 = call <vilib>:"Clear Errors.vi"("error in (no error)"=w73, "specific error code to clear (0: all)"=w72) -> ("error out"=w71:errorcluster)  [unwired: 4 in, 1 out]
  }
  "Loop data out" <- w57
  "Session properties out" <- w56
  "Index out" <- w44
  n520 = Unregister For Events(event registration refnum=w55, error in=w54) -> (error out=w7:errorcluster)
  n521 = Destroy User Event(user event=w5, error in=w7) -> (error out=w6:errorcluster)
  n522 = Destroy User Event(user event=w27, error in=w6) -> (error out=w30:errorcluster)
  n523 = Destroy User Event(user event=w35, error in=w30) -> (error out=w46:errorcluster)
  n524 = Destroy User Event(user event=w22, error in=w46) -> (error out=→"Error Out":errorcluster)
  "Workspace out" <- "Workspace base"
  "Actual file out" <- "Actual file"
